vi "HMI CSE1.vi"() -> ()   [LabVIEW 2010]
uses:
  <vilib>/addons/Simulation Interface/_sitctls/sit Indicator Info.ctl
  <vilib>/addons/Simulation Interface/_sitctls/sit Indicator Type.ctl
  <vilib>/addons/Simulation Interface/_sitctls/sit Client Meta Info (v3).ctl
  <vilib>/addons/Simulation Interface/_sitctls/sit MDL Line Item Info.ctl
  <vilib>/addons/Simulation Interface/_sitctls/sit MDL Line Type.ctl
  <vilib>/addons/Simulation Interface/_sitctls/sit Details Settings.ctl
  <vilib>/addons/Simulation Interface/_sitctls/sit Execution Host.ctl
  <vilib>/addons/Simulation Interface/_sitctls/SIT Sim State.ctl
  <vilib>/Utility/inputDevices.llb/closeJoystick.vi
  <vilib>/Utility/inputDevices.llb/joystickAcquire.vi
  <vilib>/addons/Simulation Interface/_sitclient.llb/NI_SIT_sitclient.lvlib
  <vilib>/addons/Simulation Interface/_sitctls/NI_SIT_sitctls.lvlib
  <vilib>/ptbypt/NI_PtbyPt.lvlib
  <vilib>/picture/3D Picture Control/NI_3D Picture Control.lvlib
panel:
  out "Navigation eta yaw":dbl
  out "Navigation eta sway":dbl
  out "Navigation eta surge":dbl
  out "Plant u5":dbl
  out "Plant u4":dbl
  out "Plant u3":dbl
  out "Plant u2":dbl
  out "Plant u1":dbl
  out "DP eta Psi deg":dbl
  out "DP eta E":dbl
  out "DP eta N":dbl
  out "DP eta_d Psi deg":dbl
  out "DP eta_d E":dbl
  out "DP eta_d N":dbl
  in  "Enabler Nothing":bool
  in  "Enable Linear Simulator":bool
  in  "Control Input Selector":enum32{"OK Button 4", "OK Button 5"}(radio)
  in  "MODE":T1(radio)=enum."OK Button 4"
  in  "Enable CSE1 actuator":bool
  in  "SIT_RVE":bool
  in  "SIT_Remap":bool
  in  "SIT_Details":bool
  in  "SIT_Stop":bool
  in  "SIT_Pause":bool
  in  "SIT_Run":bool
  in  "SIT_stopVI":bool
  out "SIT_Status":string
  in  "Tab Front Pannel":T2(tab)
  out "Port VSP Direction":dbl(knob) scale=0.0..360.0
  out "Starboard VSP Direction":dbl(knob) scale=0.0..360.0
  in  "Precision  VSP Speed limit":dbl
  in  "Precision u5":dbl
  in  "Precision u4":dbl
  in  "Precision u3":dbl
  in  "Precision u2":dbl
  in  "Precision u1":dbl
  out "Slide BT red":dbl(slide)
  out "Slide BT green":dbl(slide) scale=0.0..1.0
  out "Magnitude Pitch Starboard VSP":dbl(knob) scale=0.0..1.0
  out "Magnitude Pitch Port VSP":dbl(knob) scale=0.0..1.0
  out "Direction Starboard VSP":cluster{dbl, dbl}(knob)={0.0, -90.87174020086496} scale=180.0..-180.0
  out "Direction Port VSP":cluster{dbl, dbl}(knob)={0.0, 56.36157481708119} scale=180.0..-180.0
  in  "Precision BT Power limit":dbl
  in  "VSP Slide Speed":dbl(slide) min=-1.0 max=1.0 step=0.05 scale=-1.0..1.0 scale format="%#_2g"
  in  "BT Slide Power Limiter":dbl(slide) min=0.0 max=1.0 step=0.1 scale=-1.0..1.0
  in  "Left Y":dbl(slide) scale=-35860.0..35860.0
  in  "Left X":dbl(slide) scale=-35860.0..35860.0
  in  "Right X":dbl(slide) scale=-35860.0..35860.0
  in  "Right Y":dbl(slide) scale=-35860.0..35860.0
  out "Servo Battery":dbl(knob) scale=0.0..8.0
  out "Bowthruster Battery":dbl(knob) scale=0.0..8.0
  out "Main Battery":dbl(knob) scale=0.0..18.0
  out "Left Joystick":bool
  out "Right Joystick":bool
  out "Direction Up":bool
  out "Direction Right":bool
  out "Direction Down":bool
  out "Direction Left":bool
  out "L2 Button":bool
  out "R2 Button":bool
  out "Triangle Button":bool
  out "Circle Button":bool
  out "X Button":bool
  out "Square Button":bool
  out "Joystick Info":T3(array[cluster])
  in  "L2":sgl
  in  "R2":sgl
  out "Plot s":waveform(dbl)[](graph)
  out "Plot q_y":waveform(dbl)[](graph)
  out "Plot q_x":waveform(dbl)[](graph)
  in  "Tab Path":enum32{"Path", "Page 2"}(tab)
  in  "Enable path guidance":bool
  in  "u_d [m/s]":dbl
  out "Path psi_d":dbl
  out "Path y_d":dbl
  out "Path x_d":dbl
  in  "Show Path Marker":bool
  in  "my":dbl
  in  "Delta":dbl
  in  "x_2":dbl
  in  "y_2":dbl
  in  "x_1":dbl
  in  "y_1":dbl
  in  "Tab Plants":enum32{"eta", "Qualisys", "Linear Simulator"}(tab)
  in  "Tab eta":enum32{"Navigation output", "Qualisys"}(tab)
  out "Iceberg yaw":dbl
  out "Iceberg pitch":dbl
  out "Iceberg roll":dbl
  out "Iceberg z-position":dbl
  out "Iceberg y-position":dbl
  out "Iceberg x-position":dbl
  out "CSE1 yaw [rad]":dbl
  out "CSE1 pitch [rad]":dbl
  out "CSE1 roll [rad]":dbl
  out "CSE1 z-position [m]":dbl
  out "CSE1 y-position [m]":dbl
  out "CSE1 x-position [m]":dbl
  out "QS yaw [rad]":dbl
  out "QS pitch [rad]":dbl
  out "QS roll [rad]":dbl
  out "QS z-position [m]":dbl
  out "QS y-position [m]":dbl
  out "QS x-position [m]":dbl
  in  "Show CSEI":bool
  in  "Show Iceberg":bool
  out "QTM In9":dbl
  out "QTM In8":dbl
  out "QTM In7":dbl
  out "QTM In6":dbl
  out "QTM In5":dbl
  out "QTM In4":dbl
  out "QTM In3":dbl
  out "QTM In2":dbl
  out "QTM In1":dbl
  out "LS nu_yaw_hil":dbl
  out "LS nu_sway_hil":dbl
  out "LS nu_surge_hil":dbl
  out "LS etadot_yaw_hil":dbl
  out "LS etadot_sway_hil":dbl
  out "LS etadot_surge_hil":dbl
  out "LS eta_yaw_hil":dbl
  out "LS eta_sway_hil":dbl
  out "LS  eta_surge_hil":dbl
  in  "LS r_0":dbl
  in  "LS v_0":dbl
  in  "LS u_0":dbl
  in  "LS psi_0":dbl
  in  "LS y_0":dbl
  in  "LS x_0":dbl
  in  "Button Reset Linear Simulator Integrator":bool
  in  "Reset Linear Simulator integrator":dbl
  in  "Tab Control system":T4(tab)
  in  "DP Wave Filter":bool
  in  "DP eta_d LPF":bool
  in  "DP K_d Scale":dbl(slide) min=0.0 max=5.0 step=0.25 scale=0.0..5.0
  in  "DP K_i Scale":dbl(slide) min=0.0 max=5.0 step=0.25 scale=0.0..5.0
  in  "DP K_p Scale":dbl(slide) min=0.0 max=10.0 step=0.5 scale=0.0..10.0
  in  "DP eta_d_N [m]":dbl
  in  "DP eta_d_E [m]":dbl
  in  "Button Reset DP Integrator.":bool
  in  "DP eta_d_Psi [deg]":dbl(knob) scale=0.0..360.0 scale format="%#.3p"
  out "Ind eta_d_Psi [rad]":dbl format="%#_2g"
  in  "Reset DP Integrator":dbl
  in  "Show DP Marker":bool
  in  "LgV2 q_y0":dbl
  in  "LgV2 q_x0":dbl
  in  "LgV2 s_0":dbl
  in  "LgV2 lambda":dbl
  in  "LgV2 Gamma_q Sway":dbl
  in  "LgV2 Gamma_q Surge":dbl
  in  "LgV2 K_d yaw":dbl
  in  "LgV2 K_d Sway":dbl
  in  "LgV2 K_d Surge":dbl
  in  "LgV2 K_i yaw":dbl
  in  "LgV2 K_i Sway":dbl
  in  "LgV2 K_i Surge":dbl
  in  "LgV2 K_p yaw":dbl
  in  "LgV2 K_p Sway":dbl
  in  "LgV2 K_p Surge":dbl
  in  "LgV2 kappa_1":dbl
  in  "Button Reset LgV2 q":bool
  in  "Button Reset LgV2 s":bool
  in  "Reset LgV2 q":dbl
  in  "Reset LgV2 s":dbl
  in  "NLPID q_y0":dbl
  in  "NLPID q_x0":dbl
  in  "NLPID s_0":dbl
  in  "NLPID lambda":dbl
  in  "NLPID Gamma_q Sway":dbl
  in  "NLPID Gamma_q Surge":dbl
  in  "NLPID K_d yaw":dbl
  in  "NLPID K_d Sway":dbl
  in  "NLPID K_d Surge":dbl
  in  "NLPID K_i yaw":dbl
  in  "NLPID K_i Sway":dbl
  in  "NLPID K_i Surge":dbl
  in  "NLPID K_p yaw":dbl
  in  "NLPID K_p Sway":dbl
  in  "NLPID K_p Surge":dbl
  in  "Button Reset NLPID s":bool
  in  "Button Reset NLPID q":bool
  in  "Reset NLPID s":dbl
  in  "Reset NLPID q":dbl
  out "3D Picture":refnum<vi>(3d-picture)
  in  "Tab Reg plots":enum32{"DP", "Page 2"}(tab)
  out "DP Reponse N":cluster{"Value":dbl, "Value":dbl}(graph)
  out "DP Error N":waveform(dbl)[](graph)
  out "DP Error E":waveform(dbl)[](graph)
  out "DP Error Psi":waveform(dbl)[](graph)
  out "DP Reponse Psi":cluster{"Value":dbl, "Value":dbl}(graph)
  out "DP Response E":cluster{"Value":dbl, "Value":dbl}(graph)
  in  "Tab Command":enum32{"DP", "Page 2"}(tab)
  out "DP tau surge":waveform(dbl)[](graph)
  out "DP tau sway":waveform(dbl)[](graph)
  out "DP tau yaw":waveform(dbl)[](graph)
  out "DP u_1":waveform(dbl)[](graph)
  out "DP u_2":waveform(dbl)[](graph)
  out "DP u_3":waveform(dbl)[](graph)
  out "DP u_4":waveform(dbl)[](graph)
  out "DP u_5":waveform(dbl)[](graph)
  in  "SIT_Meta_Info":T5
  in  "SIT_Indicator_Indices":T10[](array[typedef])=[{"Indicator Index"=0, "Number of Signals"=1, "Indicator Type"=enum."Knob"}, {"Indicator Index"=-1, "Number of Signals"=0, "Indicator Type"=enum."Digital"}, {"Indicator Index"=-1, "Number of Signals"=0, "Indicator Type"=enum."Digital"}, {"Indicator Index"=3, "Number of Signals"=1, "Indicator Type"=enum."Digital"}, {"Indicator Index"=4, "Number of Signals"=1, "Indicator Type"=enum."Digital"}, {"Indicator Index"=5, "Number of Signals"=1, "Indicator Type"=enum."Digital"}, {"Indicator Index"=-1, "Number of Signals"=0, "Indicator Type"=enum."Digital"}, {"Indicator Index"=7, "Number of Signals"=1, "Indicator Type"=enum."WaveformChart"}, {"Indicator Index"=8, "Number of Signals"=1, "Indicator Type"=enum."WaveformChart"}, {"Indicator Index"=9, "Number of Signals"=1, "Indicator Type"=enum."WaveformChart"}, {"Indicator Index"=10, "Number of Signals"=1, "Indicator Type"=enum."Digital"}, {"Indicator Index"=11, "Number of Signals"=1, "Indicator Type"=enum."Digital"}, {"Indicator Index"=12, "Number of Signals"=1, "Indicator Type"=enum."Digital"}, {"Indicator Index"=13, "Number of Signals"=1, "Indicator Type"=enum."Digital"}, {"Indicator Index"=14, "Number of Signals"=1, "Indicator Type"=enum."Digital"}, {"Indicator Index"=15, "Number of Signals"=1, "Indicator Type"=enum."Digital"}, {"Indicator Index"=16, "Number of Signals"=1, "Indicator Type"=enum."WaveformChart"}, {"Indicator Index"=17, "Number of Signals"=1, "Indicator Type"=enum."WaveformChart"}, {"Indicator Index"=18, "Number of Signals"=1, "Indicator Type"=enum."WaveformChart"}, {"Indicator Index"=19, "Number of Signals"=1, "Indicator Type"=enum."WaveformChart"}, {"Indicator Index"=20, "Number of Signals"=1, "Indicator Type"=enum."WaveformChart"}, {"Indicator Index"=21, "Number of Signals"=1, "Indicator Type"=enum."WaveformChart"}, {"Indicator Index"=22, "Number of Signals"=1, "Indicator Type"=enum."WaveformChart"}, {"Indicator Index"=23, "Number of Signals"=1, "Indicator Type"=enum."WaveformChart"}, {"Indicator Index"=-1, "Number of Signals"=0, "Indicator Type"=enum."Knob"}, {"Indicator Index"=-1, "Number of Signals"=0, "Indicator Type"=enum."Knob"}, {"Indicator Index"=-1, "Number of Signals"=0, "Indicator Type"=enum."Digital"}, {"Indicator Index"=-1, "Number of Signals"=0, "Indicator Type"=enum."Digital"}, {"Indicator Index"=28, "Number of Signals"=1, "Indicator Type"=enum."Digital"}, {"Indicator Index"=29, "Number of Signals"=1, "Indicator Type"=enum."Digital"}, {"Indicator Index"=30, "Number of Signals"=1, "Indicator Type"=enum."Digital"}, {"Indicator Index"=-1, "Number of Signals"=0, "Indicator Type"=enum."Digital"}, {"Indicator Index"=32, "Number of Signals"=1, "Indicator Type"=enum."Digital"}, {"Indicator Index"=33, "Number of Signals"=1, "Indicator Type"=enum."Digital"}, {"Indicator Index"=34, "Number of Signals"=1, "Indicator Type"=enum."Digital"}, {"Indicator Index"=35, "Number of Signals"=1, "Indicator Type"=enum."Digital"}, {"Indicator Index"=36, "Number of Signals"=1, "Indicator Type"=enum."Digital"}, {"Indicator Index"=37, "Number of Signals"=1, "Indicator Type"=enum."Digital"}, {"Indicator Index"=38, "Number of Signals"=1, "Indicator Type"=enum."Digital"}, {"Indicator Index"=39, "Number of Signals"=1, "Indicator Type"=enum."Digital"}, {"Indicator Index"=40, "Number of Signals"=1, "Indicator Type"=enum."Digital"}, {"Indicator Index"=41, "Number of Signals"=1, "Indicator Type"=enum."Knob"}, {"Indicator Index"=42, "Number of Signals"=1, "Indicator Type"=enum."Knob"}, {"Indicator Index"=43, "Number of Signals"=1, "Indicator Type"=enum."Knob"}, {"Indicator Index"=44, "Number of Signals"=1, "Indicator Type"=enum."Digital"}, {"Indicator Index"=45, "Number of Signals"=1, "Indicator Type"=enum."Digital"}, {"Indicator Index"=46, "Number of Signals"=1, "Indicator Type"=enum."Digital"}, {"Indicator Index"=47, "Number of Signals"=1, "Indicator Type"=enum."Digital"}, {"Indicator Index"=48, "Number of Signals"=1, "Indicator Type"=enum."Digital"}, {"Indicator Index"=49, "Number of Signals"=1, "Indicator Type"=enum."Digital"}, {"Indicator Index"=50, "Number of Signals"=1, "Indicator Type"=enum."Digital"}, {"Indicator Index"=51, "Number of Signals"=1, "Indicator Type"=enum."Digital"}, {"Indicator Index"=52, "Number of Signals"=1, "Indicator Type"=enum."Digital"}, {"Indicator Index"=53, "Number of Signals"=1, "Indicator Type"=enum."Digital"}, {"Indicator Index"=54, "Number of Signals"=1, "Indicator Type"=enum."Digital"}, {"Indicator Index"=55, "Number of Signals"=1, "Indicator Type"=enum."WaveformChart"}, {"Indicator Index"=56, "Number of Signals"=1, "Indicator Type"=enum."WaveformChart"}, {"Indicator Index"=57, "Number of Signals"=1, "Indicator Type"=enum."WaveformChart"}, {"Indicator Index"=58, "Number of Signals"=1, "Indicator Type"=enum."Knob"}, {"Indicator Index"=59, "Number of Signals"=1, "Indicator Type"=enum."Digital"}, {"Indicator Index"=60, "Number of Signals"=1, "Indicator Type"=enum."Digital"}, {"Indicator Index"=61, "Number of Signals"=1, "Indicator Type"=enum."Digital"}, {"Indicator Index"=62, "Number of Signals"=1, "Indicator Type"=enum."Digital"}, {"Indicator Index"=63, "Number of Signals"=1, "Indicator Type"=enum."Digital"}, {"Indicator Index"=64, "Number of Signals"=1, "Indicator Type"=enum."Digital"}, {"Indicator Index"=65, "Number of Signals"=1, "Indicator Type"=enum."Digital"}, {"Indicator Index"=66, "Number of Signals"=1, "Indicator Type"=enum."Digital"}, {"Indicator Index"=67, "Number of Signals"=1, "Indicator Type"=enum."Digital"}, {"Indicator Index"=68, "Number of Signals"=1, "Indicator Type"=enum."Digital"}, {"Indicator Index"=69, "Number of Signals"=1, "Indicator Type"=enum."Digital"}, {"Indicator Index"=70, "Number of Signals"=1, "Indicator Type"=enum."Digital"}, {"Indicator Index"=71, "Number of Signals"=1, "Indicator Type"=enum."Digital"}, {"Indicator Index"=72, "Number of Signals"=1, "Indicator Type"=enum."Digital"}, {"Indicator Index"=73, "Number of Signals"=1, "Indicator Type"=enum."Digital"}, {"Indicator Index"=74, "Number of Signals"=1, "Indicator Type"=enum."Knob"}, {"Indicator Index"=75, "Number of Signals"=1, "Indicator Type"=enum."Slide"}, {"Indicator Index"=76, "Number of Signals"=1, "Indicator Type"=enum."Slide"}, {"Indicator Index"=77, "Number of Signals"=1, "Indicator Type"=enum."Knob"}]
  # "MODE"
  # "Controller Input Selector"
  # "TARGET"
  # "Model Controls"
  # "Precision control"
  # "Bowthruster"
  # "VSP Speed"
  # "VSP speed = 1\n\nStarboard VSP\nMax Speed  ClockWise\n\nPort VSP \nMax Speed CounterClockWise"
  # "VSP Speed = -1\n\nStarboard VSP \nMax Speed CounterClockWise\n\nPort VSP\nMax Speed ClockWise"
  # "Port VSP pitch"
  # "Starboard VSP pitch"
  # "Bow Thruster Power Limit"
  # "Max Power"
  # "Max Power"
  # "No Power"
  # "PS3 Joysticks"
  # "Increase BT power limit"
  # "Increase VSP speed"
  # "Decrease BT power limit"
  # "Decrease VSP speed"
  # "Port VSP\n(surge/sway force setpoint)"
  # "Starboard VSP"
  # "C/S Enterprise I"
  # "Toggle visibility"
  # "Iceberg"
  # "Toggle visibility"
  # "Initial eta"
  # "Initial nu"
  # "DP controller gains"
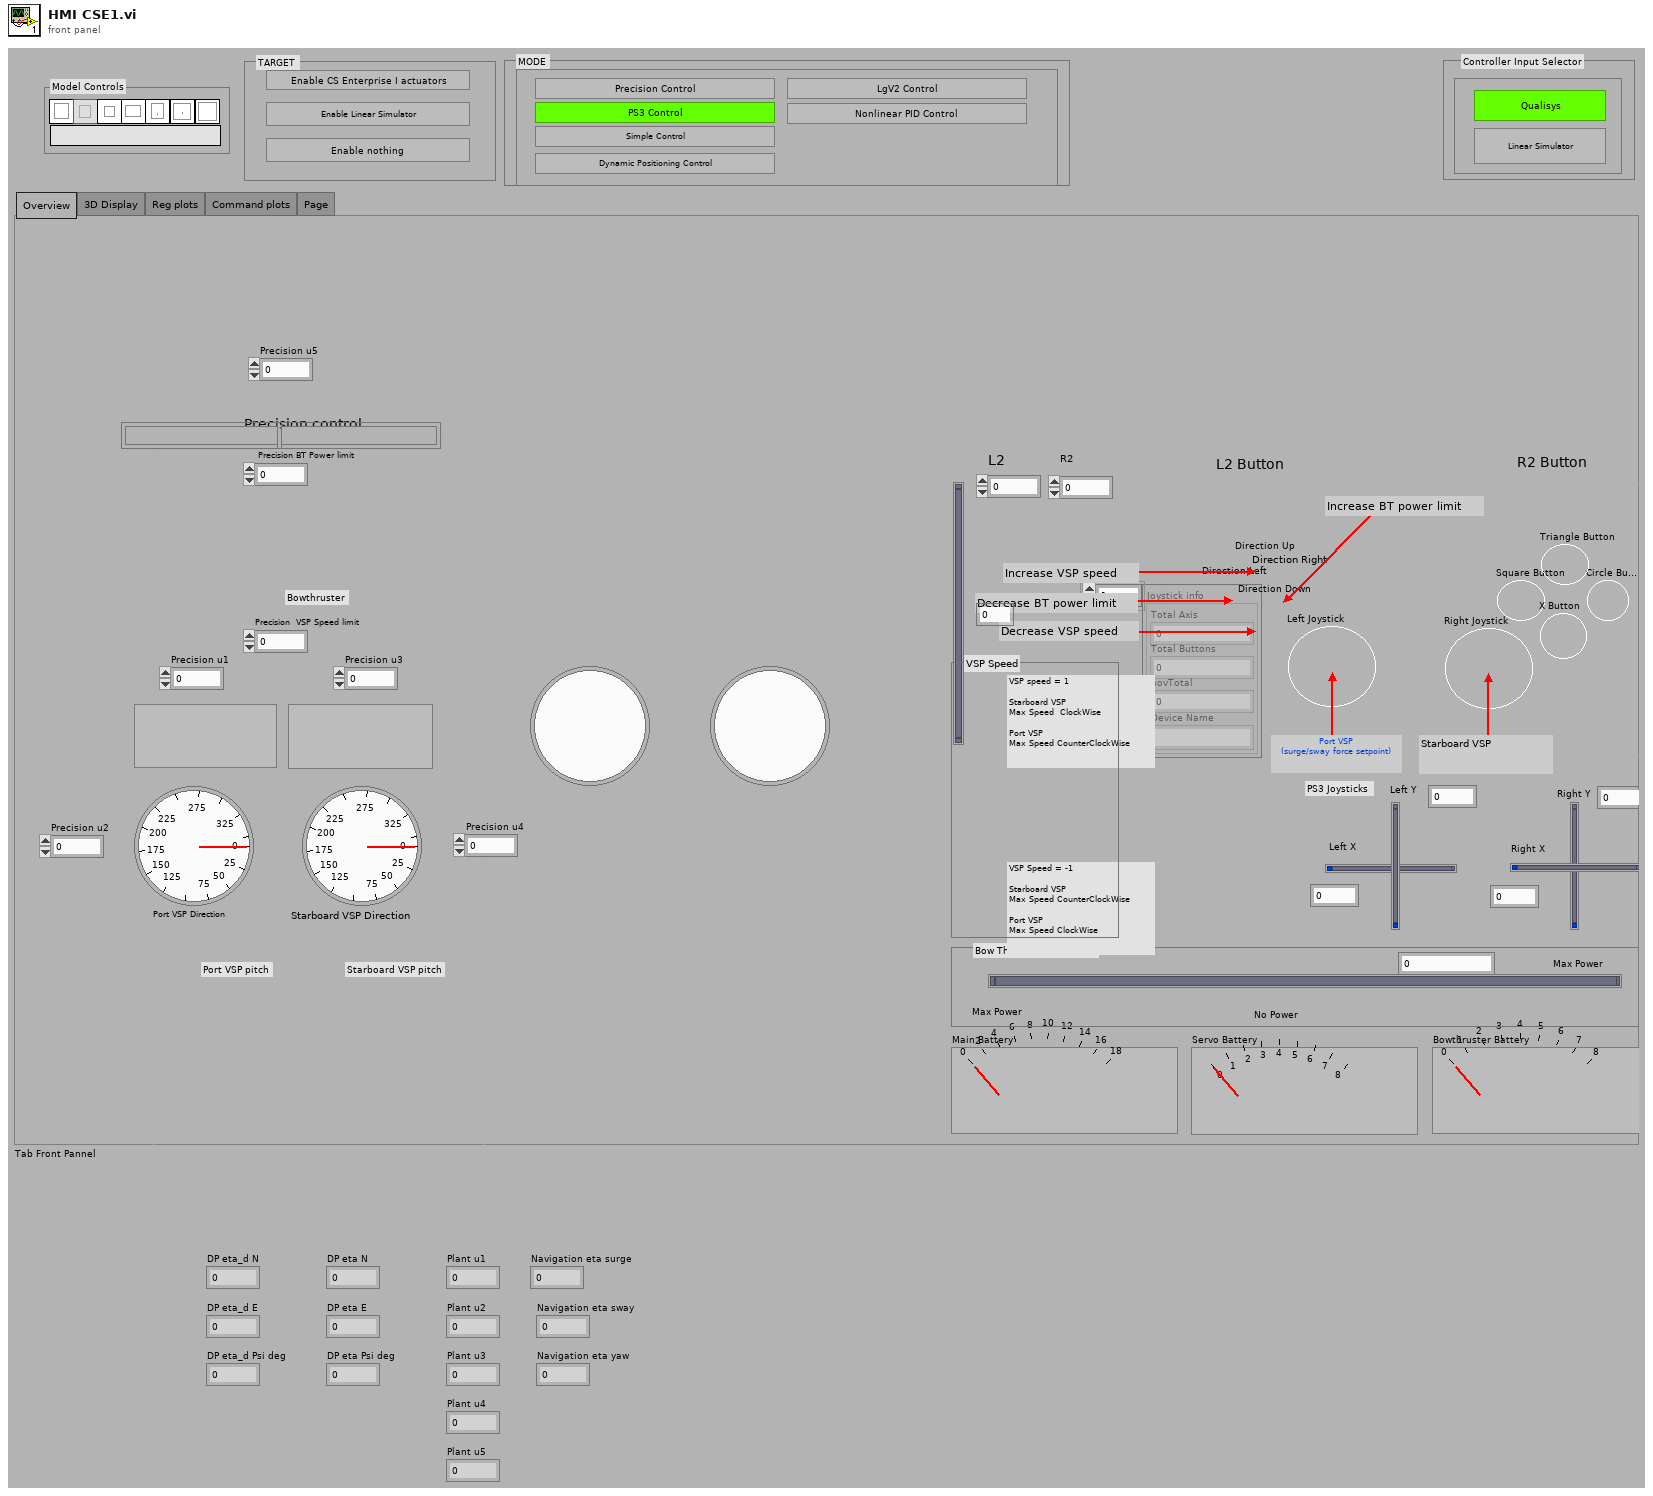
[diagram p1: front panel]
types:
  T1 = enum32{"Radio Selection 4", "OK Button 4", "OK Button 5", "OK Button 6", "Radio Selection 5", "Radio Selection 6"}
  T2 = enum32{"Overview", "3D Display", "Reg plots", "Command plots", "Page"}
  T3 = cluster{"Total Axis":u32, "Total Buttons":u32, "povTotal":u32, "Device Name":string}[]
  T4 = enum32{"DP Control", "LgV2 Control", "NLPID control"}
  T5 = typedef "NI_SIT_sitctls.lvlib/sit Client Meta Info (v3).ctl" = cluster{"Simulation IP":string, "Target IP":string, "Host Port":u16, "Model DLL Path":path, "Model File Path":path, "Model Name":string, "Param Tree Info ":T6[], "Signal Tree Info":T6[], "Details Settings":T8, "Client Name":string, "Stored Model Checksum":string, "Buffer Sizes":cluster{"number of signals":u32, "circular buffer size":u32, "num data points":u32}, "Execution Host":T9, "Project Dir":path, "Last MDL":path}
  T6 = typedef "NI_SIT_sitctls.lvlib/sit MDL Line Item Info.ctl" = cluster{"Line Type":T7, "Section Type":string, "Name":string, "Value":string, "Owner Index":i32, "Tree Tag":string, "Child Indices":i32[], "Expanded?":bool, "Destination Block Info":string[]}
  T7 = typedef "NI_SIT_sitctls.lvlib/sit MDL Line Type.ctl" = enum16{"Section Head", "Parameter", "Section End", "Comment"}
  T8 = typedef "NI_SIT_sitctls.lvlib/sit Details Settings.ctl" = cluster{"Halt on Task Overrun?":bool, "Halt on Lost Data?":bool, "Signal Decimation":i32, "Autoscale":bool}
  T9 = typedef "NI_SIT_sitctls.lvlib/sit Execution Host.ctl" = enum32{"Simulation Environment", "RT Target", "Local Driver"}
  T10 = typedef "NI_SIT_sitctls.lvlib/sit Indicator Info.ctl" = cluster{"Indicator Index":i32, "Number of Signals":i32, "Indicator Type":T11}
  T11 = typedef "NI_SIT_sitctls.lvlib/sit Indicator Type.ctl" = enum32{"xxx1", "xxx2", "xxx3", "Generic   ", "Decoration", "Text", "xControl", "ColorBox", "Boolean", "RefNum", "Variant", "Path", "ListBox", "Table", "Array", "Picture", "ActiveXContainer", "Numeric", "Digital", "NamedNumeric", "ColorRamp", "Slide", "GraphOrChart", "WaveformChart", "WaveformGraph", "IntensityChart", "xxx4", "xxx5", "xxx6", "xxx7", "Cluster", "Panel", "Knob", "NumWithScale", "Ring", "Enum", "GObject", "Plot", "Cursor", "NumericText", "Scale", "ColorScale", "GraphScale", "ColorGraphScale", "TypedRefNum", "OldKnobScale", "MCListbox", "WaveformData", "BVTag", "DAQName", "VISAName", "IVIName", "SlideScale"}
  T12 = cluster{"Red":sgl, "Green":sgl, "Blue":sgl, "Alpha":sgl}
  T13 = cluster{"axes total":u32, "buttons total":u32, "pov total":u32, "device name":string}[]
  T14 = typedef "NI_SIT_sitctls.lvlib/sit TCP Conn and Queue.ctl" = cluster{"TCP Connection":refnum<k5>, "Data Queue":refnum<queue>, "Execution Host":T9}
  T15 = typedef "NI_SIT_sitctls.lvlib/sit Client Op Refs.ctl" = cluster{"Conn and Queue":T14, "RunPauseStop Refs":refnum<vi>[], "Control Refs":refnum<vi>[], "Indicator Refs":refnum<vi>[], "Param Info":T16[], "State Queue":refnum<queue>, "Don't Modify Scales?":bool, "Param Info Needs Init?":bool}
  T16 = typedef "NI_SIT_sitctls.lvlib/SIT param info.ctl" = cluster{"paramidx":i32, "ID":string, "paramname":string, "dattype":i32, "Dimensions":i32[], "value":dbl[]}
  T17 = typedef "NI_SIT_sitctls.lvlib/SIT Sim State.ctl" = enum8{"Default", "Idle", "Running", "Paused", "Stopped", "Error"}
  T18 = cluster{"X axis":i32, "Y axis":i32, "Z axis":i32, "X axis rotation":i32, "Y axis rotation":i32, "Z axis rotation":i32, "U axis":i32, "V axis":i32}
  T19 = cluster{"button 1":bool, "button 2":bool, "button 3":bool, "button 4":bool, "button 5":bool, "button 6":bool, "button 7":bool, "button 8":bool, "button 9":bool, "button 10":bool, "button 11":bool, "button 12":bool, "button 13":bool, "button 14":bool, "button 15":bool, "button 16":bool, "button 17":bool, "button 18":bool, "button 19":bool, "button 20":bool, "button 21":bool, "button 22":bool, "button 23":bool, "button 24":bool, "button 25":bool, "button 26":bool, "button 27":bool, "button 28":bool, "button 29":bool, "button 30":bool, "button 31":bool, "button 32":bool}
  T20 = cluster{"pov 1":i32, "pov 2":i32, "pov 3":i32, "pov 4":i32}
  T21 = cluster{"DP eta_d_N [m]":dbl, i32, "DP eta_d_E [m]":dbl}
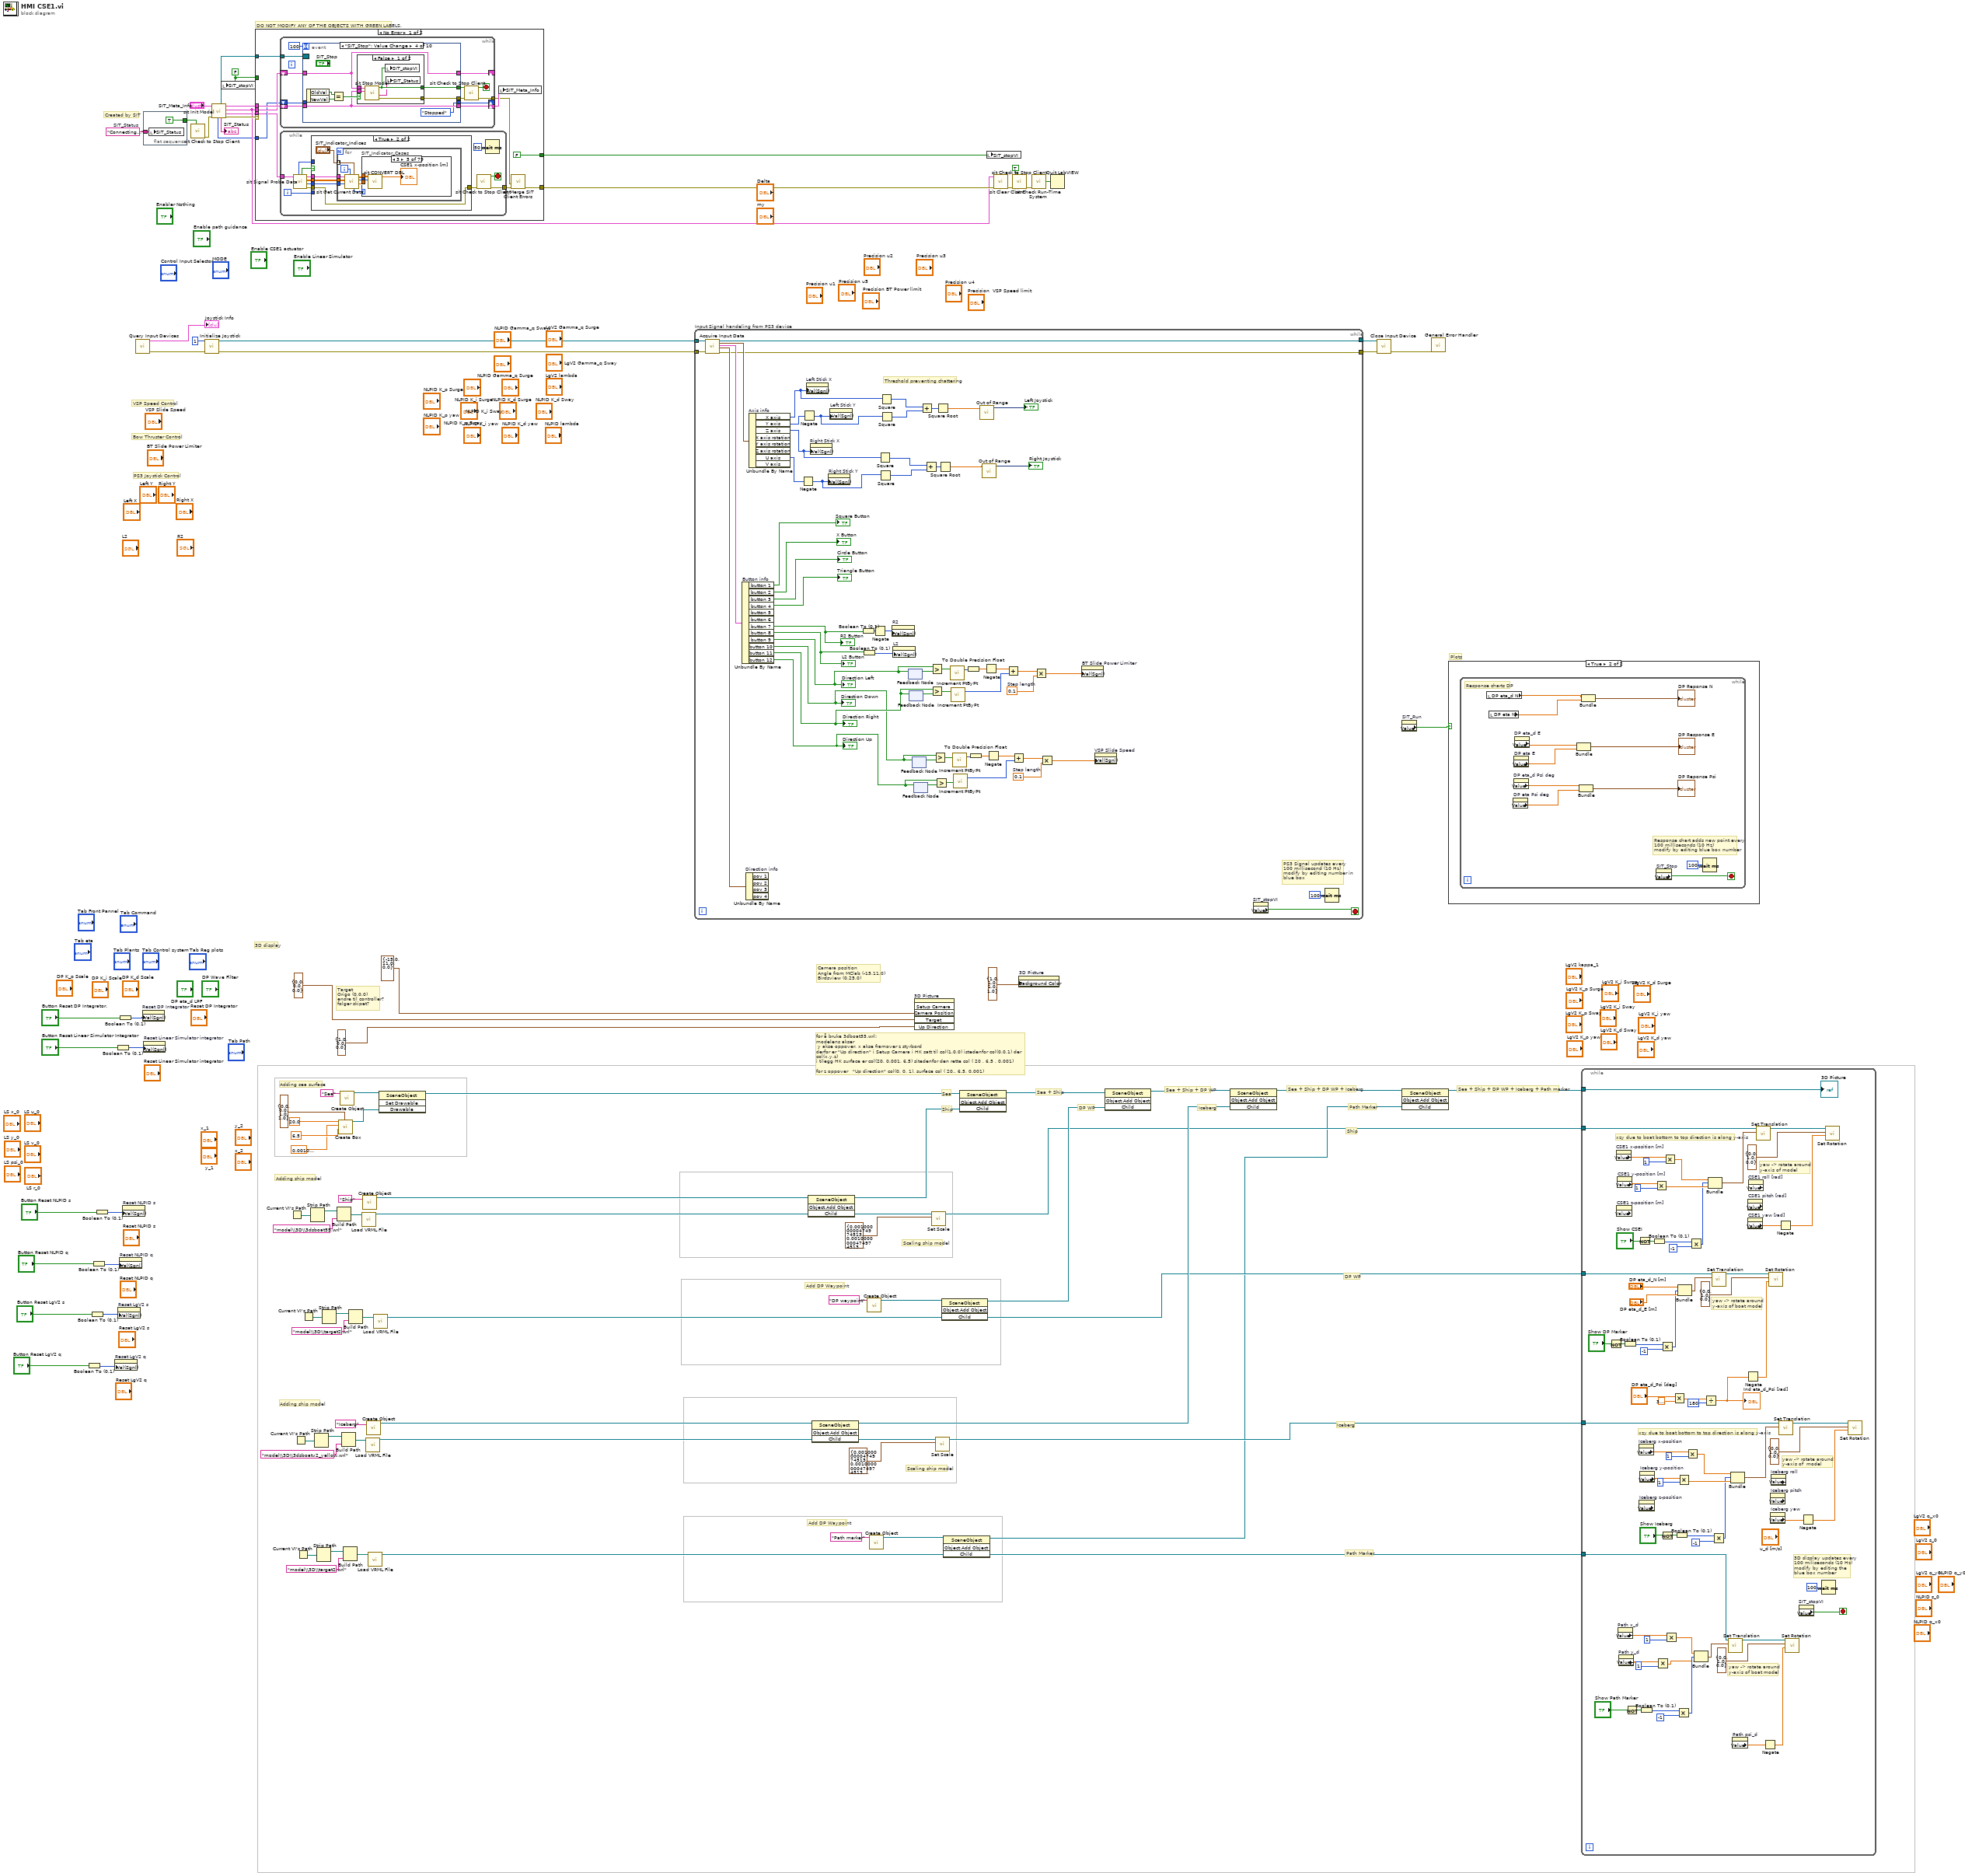
[diagram p0: block diagram]
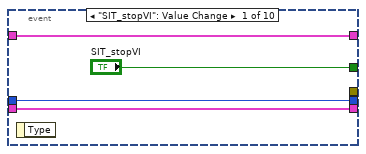
[diagram p3: hidden frame]
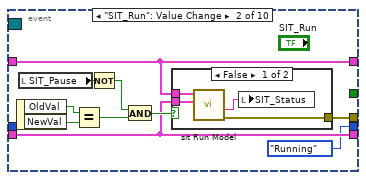
[diagram p4: hidden frame]
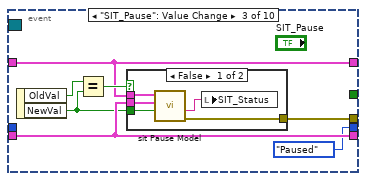
[diagram p6: hidden frame]
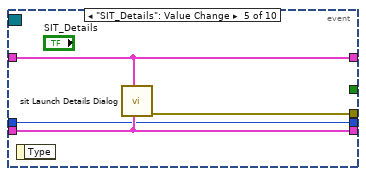
[diagram p9: hidden frame]
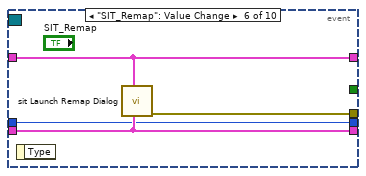
[diagram p10: hidden frame]
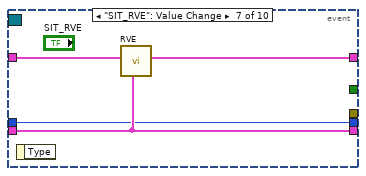
[diagram p11: hidden frame]
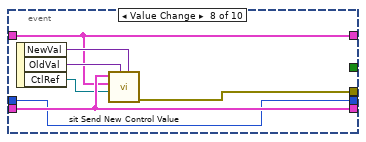
[diagram p12: hidden frame]
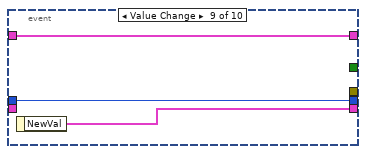
[diagram p13: hidden frame]
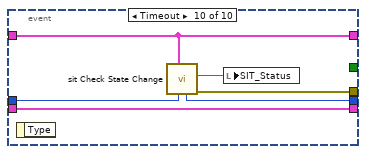
[diagram p14: hidden frame]
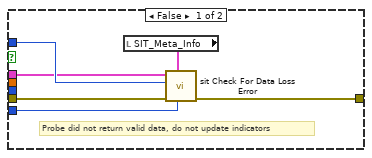
[diagram p15: hidden frame]
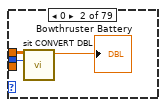
[diagram p17: hidden frame]
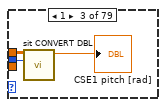
[diagram p18: hidden frame]
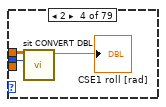
[diagram p19: hidden frame]
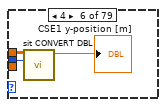
[diagram p20: hidden frame]
diagram:
  w80 = "Connecting..."  # SIT_Status
  w85 = FALSE
  # "Path Marker"
  # "Path Marker"
  # "Sea + Ship + DP WP + Iceberg + Path marker"
  # "Add DP Waypoint"
  # "Plots"
  # "Iceberg"
  # "Iceberg"
  # "Sea + Ship + DP WP + Iceberg"
  # "Scaling ship model"
  # "Adding ship model"
  # "DP WP"
  # "Ship"
  # "3D display"
  # "DP WP"
  # "Target\nOrigo (0,0,0)\nendre til controller?\nfølger skipet?"
  # "Scaling ship model"
  # "Camera position\nAngle from MClab (-15,11,0)\nBirdsview (0,25,0)"
  # "Add DP Waypoint"
  # "Sea + Ship + DP WP"
  # "for å bruke 3dboat55.wrl:\nmodelens akser\n y akse oppover, x akse framover z styrbord\nderfor er \"Up direction\" i Setup Camera i HK satt til col(1,0,0) istedenfor col(0,0,1) der col(x,y,z)\ni tilegg HK surface er col(20, 0.001, 6.5) sitedenfor den rette col ( 20 , 6.5 , 0.001) \n\nfor z oppover   \"Up direction\" col(0, 0, 1), surface col ( 20., 6.5, 0.001)"
  # "Sea + Ship"
  # "Ship"
  # "Sea"
  # "Adding sea surface"
  # "Adding ship model"
  # "VSP Speed Control"
  # "Bow Thruster Control"
  # "Created by SIT"
  # "PS3 Joystick Control"
  # "DO NOT MODIFY ANY OF THE OBJECTS WITH GREEN LABELS."
  n1 = Boolean To (0,1)(Boolean="Button Reset LgV2 q") -> (0, 1=w1:i16)
  n2 = Boolean To (0,1)(Boolean="Button Reset LgV2 s") -> (0, 1=w3:i16)
  n3 = Boolean To (0,1)(Boolean="Button Reset NLPID q") -> (0, 1=w5:i16)
  n4 = Boolean To (0,1)(Boolean="Button Reset NLPID s") -> (0, 1=w7:i16)
  n5 = property on="Reset LgV2 q" class="DigNum (strict)"("Val(Sgnl)"=w1) -> ()  [unwired: 2 in, 2 out]
  n6 = Boolean To (0,1)(Boolean="Button Reset Linear Simulator Integrator") -> (0, 1=w23:i16)
  n7 = Boolean To (0,1)(Boolean="Button Reset DP Integrator.") -> (0, 1=w21:i16)
  n8 = property on="Reset LgV2 s" class="DigNum (strict)"("Val(Sgnl)"=w3) -> ()  [unwired: 2 in, 2 out]
  n9 = property on="Reset NLPID q" class="DigNum (strict)"("Val(Sgnl)"=w5) -> ()  [unwired: 2 in, 2 out]
  n10 = property on="Reset NLPID s" class="DigNum (strict)"("Val(Sgnl)"=w7) -> ()  [unwired: 2 in, 2 out]
  n11 = call <vilib>:"Query Input Devices.vi"() -> ("error out"=w74:errorcluster, "joystick info"=→"Joystick Info":T13)  [unwired: 8 in, 2 out]
  n12 = property on="Reset DP Integrator" class="DigNum (strict)"("Val(Sgnl)"=w21) -> ()  [unwired: 2 in, 2 out]
  n13 = flat-sequence {
    tunnel: [TRUE ("Clear Item?")] -> w89
    tunnel: w80 -> [w96]
    frame #0 {
      n14 = local write "SIT_Status"(w96) -> ()
    }
  }
  n15 = property on="Reset Linear Simulator integrator" class="DigNum (strict)"("Val(Sgnl)"=w23) -> ()  [unwired: 2 in, 2 out]
  n16 = call <vilib>:"sit Check to Stop Client.vi"("Reset Stop?"=w89) -> ("error out"=w91:errorcluster)  [unwired: 2 in, 8 out]
  n17 = call <vilib>:"Initialize Joystick.vi"("error in (no error)"=w74, "device index"=1) -> ("error out"=w76:errorcluster, "device ID"=w77:refnum<k1>)  [unwired: 8 in]
  n18 = call <vilib>:"sit Init Model.vi"("error in (no error)"=w91, "SIT_Meta_Info in"="SIT_Meta_Info") -> ("error out"=w95:errorcluster, "Conn and Queue"=w82:T14, "SIT Client Op Refs"=w86:T15, "SIT_Meta_Info out"=w93:T5, "Initial State"=→"SIT_Status":string, "Event Registration Refnum"=w94:refnum<event-registration>, "State"=w83:T17)  [unwired: 2 in, 1 out]
  n19 = local write "SIT_stopVI"(w85) -> ()
  n20 = case shown="No Error" w95 {
    selector: w95 -> [_ w484]
    tunnel: w94 -> [w107 _]
    tunnel: w93 -> [w105 w483]
    tunnel: [w101 w484] -> w90
    tunnel: w86 -> [w104 _]
    tunnel: w85 -> [_ _]
    tunnel: [FALSE _] -> w84
    tunnel: w83 -> [w99 _]
    tunnel: w82 -> [w98 _]
    frame No Error {
      n21 = while {
        tunnel: w107 -> [w119]
        tunnel: [w117] -> w100
        shift-right: [w111] -> _
        shift-left: w104 -> [w115]
        shift-right: [w118] -> w106
        shift-left: w105 -> [w116]
        shift-right: [w108] -> _
        shift-left: w99 -> [w109]
        stop <- w110 stop-if-true
        n22 = event shown="[3] \"SIT_Stop\": Value Change" {
          selector: w119 -> [_ _ _ _ _ _ _ _ _ _]
          dyn-events: _ -> [_ _ _ _ _ _ _ _ _ _]
          timeout: 100 -> [_ _ _ _ _ _ _ _ _ _]
          tunnel: ["SIT_stopVI" _ _ w154 _ _ _ _ _ _] -> w112
          tunnel: [_ w129 w141 w153 w166 w170 _ w181 _ w188] -> w113
          tunnel: w116 -> [w122 w127 w142 w155 w165 w169 w173 w180 _ w190]
          tunnel: w115 -> [w120 w128 w143 w156 w164 w167 w174 w176 w183 w189]
          tunnel: [w122 w127 w142 w155 w165 w169 w173 w180 w184 w190] -> w118
          tunnel: [w120 w128 w143 w156 w164 w167 w172 w176 w183 w189] -> w111
          tunnel: [w121 SIT_Sim_State."Running" ("State") SIT_Sim_State."Paused" ("State") SIT_Sim_State."Stopped" ("State") w163 w168 w171 w175 w182 w186] -> w108
          tunnel: w109 -> [w121 _ _ _ w163 w168 w171 w175 w182 w187]
          event "SIT_stopVI": Value Change {
            n23 = event-data() -> ()  [unwired: 2 out]
          }
          event "SIT_Run": Value Change {
            n24 = event-data() -> ("OldVal"=w125:bool, "NewVal"=w126:bool)  [unwired: 1 out]
            n25 = local read "SIT_Pause"() -> (w132:bool)
            n26 = Equal?(x=w125, y=w126) -> (x = y?=w130:bool)
            n27 = Not(x=w132) -> (.not. x?=w133:bool)
            n28 = And(x=w133, y=w130) -> (x .and. y?=w131:bool)
            n29 = case shown="False" w131 {
              tunnel: [w137 _] -> w129
              tunnel: w128 -> [w136 _]
              tunnel: w127 -> [w135 _]
              frame False {
                n30 = call <vilib>:"sit Run Model.vi"("SIT Meta Info"=w135, "SIT Client Op Refs"=w136) -> ("error out"=w137:errorcluster, "Status"=w134:string)  [unwired: 6 in, 2 out]
                n31 = local write "SIT_Status"(w134) -> ()
              }
              frame True {
                # "Ignore value change if it is\nto the same value"
              }
            }
          }
          event "SIT_Pause": Value Change {
            n32 = event-data() -> ("OldVal"=w139:bool, "NewVal"=w140:bool)  [unwired: 1 out]
            n33 = Equal?(x=w139, y=w140) -> (x = y?=w144:bool)
            n34 = case shown="False" w144 {
              tunnel: [w149 _] -> w141
              tunnel: w143 -> [w148 _]
              tunnel: w142 -> [w147 _]
              tunnel: w140 -> [w146 _]
              frame False {
                n35 = call <vilib>:"sit Pause Model.vi"("Pause Button Value"=w146, "SIT Meta Info"=w147, "SIT Client Op Refs"=w148) -> ("error out"=w149:errorcluster, "Status"=w145:string)  [unwired: 3 in, 4 out]
                n36 = local write "SIT_Status"(w145) -> ()
              }
              frame True {
                # "Ignore value change if it is\nto the same value"
              }
            }
          }
          event "SIT_Stop": Value Change {
            n37 = event-data() -> ("OldVal"=w151:bool, "NewVal"=w152:bool)  [unwired: 1 out]
            n38 = Equal?(x=w151, y=w152) -> (x = y?=w157:bool)
            n39 = case shown="False" w157 {
              tunnel: [w162 _] -> w153
              tunnel: [w159 _] -> w154
              tunnel: w155 -> [w161 _]
              tunnel: w156 -> [w160 _]
              frame False {
                n40 = call <vilib>:"sit Stop Model.vi"("SIT Meta Info"=w161, "SIT Client Op Refs"=w160) -> ("error out"=w162:errorcluster, "Status"=w158:string, "Stop VI?"=w159:bool)  [unwired: 4 in, 3 out]
                n41 = local write "SIT_stopVI"(w159) -> ()
                n42 = local write "SIT_Status"(w158) -> ()
              }
              frame True {
                # "Ignore value change if it is\nto the same value"
              }
            }
          }
          event "SIT_Details": Value Change {
            n43 = event-data() -> ()  [unwired: 2 out]
            n44 = call <vilib>:"sit Launch Details Dialog.vi"("SIT Meta Info in"=w165, "SIT Client Op Refs"=w164) -> ("error out"=w166:errorcluster)  [unwired: 1 in, 8 out]
          }
          event "SIT_Remap": Value Change {
            n45 = event-data() -> ()  [unwired: 2 out]
            n46 = call <vilib>:"sit Launch Remap Dialog.vi"("SIT Meta Info in"=w169, "SIT Client Op Refs"=w167) -> ("error out"=w170:errorcluster)  [unwired: 2 in, 7 out]
          }
          event "SIT_RVE": Value Change {
            n47 = event-data() -> ()  [unwired: 2 out]
            n48 = call <vilib>:"RVE.vi"("SIT_Meta_Info"=w173, "SIT Client Op Refs in"=w174) -> ("SIT Client Op Refs out"=w172:T15)  [unwired: 9 out]
          }
          event Value Change {
            n49 = event-data() -> ("NewVal"=w177:variant, "OldVal"=w178:variant, "CtlRef"=w179:refnum<vi>)  [unwired: 1 out]
            n50 = call <vilib>:"sit Send New Control Value.vi"("Control New Value"=w177, "Control Old Value"=w178, "Control Ref"=w179, "SIT Client Op Refs"=w176, "SIT_Meta_Info"=w180) -> ("error out"=w181:errorcluster)  [unwired: 4 in, 2 out]
          }
          event Value Change {
            n51 = event-data() -> ("NewVal"=w184:T5)  [unwired: 1 out]
          }
          event Timeout {
            n52 = event-data() -> ()  [unwired: 2 out]
            n53 = call <vilib>:"sit Check State Change.vi"("Old State in"=w187, "SIT Client Op Refs"=w189) -> ("error out"=w188:errorcluster, "Status String"=w185:string, "New State out"=w186:T17)  [unwired: 7 out]
            n54 = local write "SIT_Status"(w185) -> ()
          }
        }
        n55 = call <vilib>:"sit Check to Stop Client.vi"("error in (no error)"=w113, "User Stop?"=w112) -> ("error out"=w117:errorcluster, "Stop?"=w110:bool)  [unwired: 1 in, 7 out]
      }
      n56 = while "Read Loop" {
        tunnel: [w201] -> w102
        tunnel: w98 -> [w191]
        i -> [w198]
        stop <- w199 stop-if-true
        n57 = call <vilib>:"sit Signal Probe Data.vi"("TCP Conn and Queue"=w191) -> ("error out"=w194:errorcluster, "Dimensions"=w195:i32[], "Raw Data"=w196:dbl[][], "dup TCP Conn and Queue"=w197:T14, "Valid Data?"=w192:bool, "Options out"=w193:u32)  [unwired: 4 in, 1 out]
        n58 = case shown="True" w192 {
          tunnel: w196 -> [_ w212]
          tunnel: w195 -> [_ w211]
          tunnel: w197 -> [w204 w210]
          tunnel: w194 -> [w207 w209]
          tunnel: [w206 w209] -> w200
          tunnel: w193 -> [w208 _]
          tunnel: w198 -> [w205 _]
          frame False {
            # "Probe did not return valid data, do not update indicators"
            n59 = local read "SIT_Meta_Info"() -> (w203:T5)
            n60 = call <vilib>:"sit Check For Data Loss Error.vi"("Iteration"=w205, "SIT Meta Info"=w203, "error in (no error)"=w207, "Options"=w208, "TCP Conn and Queue"=w204) -> ("error out"=w206:errorcluster)  [unwired: 6 out]
          }
          frame True {
            n61 = for {
              tunnel: w212 -> [w222]
              tunnel: "SIT_Indicator_Indices" -> [w218] mode=indexing
              tunnel: w211 -> [w221]
              tunnel: w210 -> [w219]
              i -> [w220]
              n62 = call <vilib>:"sit Get Current Data.vi"("Indicator Index Cluster"=w218, "Iteration"=w220, "Dimensions"=w221, "Raw Data"=w222, "Conn and Queue"=w219) -> ("Timestamps"=w215:dbl[], "Last Row"=w216:i32, "Current Data"=w217:dbl[][], "Indicator Index"=w214:i32)  [unwired: 1 in, 2 out]
              n63 = case "SIT_Indicator_Cases" shown="3" w214 {
                tunnel: w217 -> [_ w225 w228 w231 w234 w237 w240 w243 w247 w252 w257 w261 w264 w267 w270 w273 w276 w280 w285 w290 w295 w300 w305 w310 w315 w318 w320 w323 w326 w329 w332 w335 w338 w341 w344 w347 w350 w353 w356 w359 w362 w365 w368 w371 w374 w377 w380 w383 w386 w389 w392 w395 w398 w401 w404 w407 w411 w416 w421 w425 w428 w431 w434 w437 w440 w443 w446 w449 w452 w455 w458 w461 w464 w467 w470 w473 w476 w479 w482]
                tunnel: w216 -> [_ w224 w227 w230 w233 w236 w239 w242 w246 w251 w256 w260 w263 w266 w269 w272 w275 w279 w284 w289 w294 w299 w304 w309 w314 w317 w319 w322 w325 w328 w331 w334 w337 w340 w343 w346 w349 w352 w355 w358 w361 w364 w367 w370 w373 w376 w379 w382 w385 w388 w391 w394 w397 w400 w403 w406 w410 w415 w420 w424 w427 w430 w433 w436 w439 w442 w445 w448 w451 w454 w457 w460 w463 w466 w469 w472 w475 w478 w481]
                tunnel: w215 -> [_ _ _ _ _ _ _ _ w245 w250 w255 _ _ _ _ _ _ w278 w283 w288 w293 w298 w303 w308 w313 _ _ _ _ _ _ _ _ _ _ _ _ _ _ _ _ _ _ _ _ _ _ _ _ _ _ _ _ _ _ _ w409 w414 w419 _ _ _ _ _ _ _ _ _ _ _ _ _ _ _ _ _ _ _ _]
                frame -1, Default {
                }
                frame 0 {
                  n64 = call <vilib>:"sit CONVERT DBL.vi"("Last Row"=w224, "Raw Data"=w225) -> ("Output"=→"Bowthruster Battery":dbl)  [unwired: 9 in]
                }
                frame 1 {
                  n65 = call <vilib>:"sit CONVERT DBL.vi"("Last Row"=w227, "Raw Data"=w228) -> ("Output"=→"CSE1 pitch [rad]":dbl)  [unwired: 9 in]
                }
                frame 2 {
                  n66 = call <vilib>:"sit CONVERT DBL.vi"("Last Row"=w230, "Raw Data"=w231) -> ("Output"=→"CSE1 roll [rad]":dbl)  [unwired: 9 in]
                }
                frame 3 {
                  n67 = call <vilib>:"sit CONVERT DBL.vi"("Last Row"=w233, "Raw Data"=w234) -> ("Output"=→"CSE1 x-position [m]":dbl)  [unwired: 9 in]
                }
                frame 4 {
                  n68 = call <vilib>:"sit CONVERT DBL.vi"("Last Row"=w236, "Raw Data"=w237) -> ("Output"=→"CSE1 y-position [m]":dbl)  [unwired: 9 in]
                }
                frame 5 {
                  n69 = call <vilib>:"sit CONVERT DBL.vi"("Last Row"=w239, "Raw Data"=w240) -> ("Output"=→"CSE1 yaw [rad]":dbl)  [unwired: 9 in]
                }
                frame 6 {
                  n70 = call <vilib>:"sit CONVERT DBL.vi"("Last Row"=w242, "Raw Data"=w243) -> ("Output"=→"CSE1 z-position [m]":dbl)  [unwired: 9 in]
                }
                frame 7 {
                  n71 = call <vilib>:"sit CONVERT WaveformChart.vi"("Timestamps"=w245, "Last Row"=w246, "Raw Data"=w247) -> ("Output"=w244:waveform(dbl)[][])  [unwired: 8 in]
                  n72 = for {
                    tunnel: w244 -> [w248] mode=indexing
                    "DP Error E" <- w248
                  }
                }
                frame 8 {
                  n73 = call <vilib>:"sit CONVERT WaveformChart.vi"("Timestamps"=w250, "Last Row"=w251, "Raw Data"=w252) -> ("Output"=w249:waveform(dbl)[][])  [unwired: 8 in]
                  n74 = for {
                    tunnel: w249 -> [w253] mode=indexing
                    "DP Error N" <- w253
                  }
                }
                frame 9 {
                  n75 = call <vilib>:"sit CONVERT WaveformChart.vi"("Timestamps"=w255, "Last Row"=w256, "Raw Data"=w257) -> ("Output"=w254:waveform(dbl)[][])  [unwired: 8 in]
                  n76 = for {
                    tunnel: w254 -> [w258] mode=indexing
                    "DP Error Psi" <- w258
                  }
                }
                frame 10 {
                  n77 = call <vilib>:"sit CONVERT DBL.vi"("Last Row"=w260, "Raw Data"=w261) -> ("Output"=→"DP eta E":dbl)  [unwired: 9 in]
                }
                frame 11 {
                  n78 = call <vilib>:"sit CONVERT DBL.vi"("Last Row"=w263, "Raw Data"=w264) -> ("Output"=→"DP eta N":dbl)  [unwired: 9 in]
                }
                frame 12 {
                  n79 = call <vilib>:"sit CONVERT DBL.vi"("Last Row"=w266, "Raw Data"=w267) -> ("Output"=→"DP eta Psi deg":dbl)  [unwired: 9 in]
                }
                frame 13 {
                  n80 = call <vilib>:"sit CONVERT DBL.vi"("Last Row"=w269, "Raw Data"=w270) -> ("Output"=→"DP eta_d E":dbl)  [unwired: 9 in]
                }
                frame 14 {
                  n81 = call <vilib>:"sit CONVERT DBL.vi"("Last Row"=w272, "Raw Data"=w273) -> ("Output"=→"DP eta_d N":dbl)  [unwired: 9 in]
                }
                frame 15 {
                  n82 = call <vilib>:"sit CONVERT DBL.vi"("Last Row"=w275, "Raw Data"=w276) -> ("Output"=→"DP eta_d Psi deg":dbl)  [unwired: 9 in]
                }
                frame 16 {
                  n83 = call <vilib>:"sit CONVERT WaveformChart.vi"("Timestamps"=w278, "Last Row"=w279, "Raw Data"=w280) -> ("Output"=w277:waveform(dbl)[][])  [unwired: 8 in]
                  n84 = for {
                    tunnel: w277 -> [w281] mode=indexing
                    "DP tau surge" <- w281
                  }
                }
                frame 17 {
                  n85 = call <vilib>:"sit CONVERT WaveformChart.vi"("Timestamps"=w283, "Last Row"=w284, "Raw Data"=w285) -> ("Output"=w282:waveform(dbl)[][])  [unwired: 8 in]
                  n86 = for {
                    tunnel: w282 -> [w286] mode=indexing
                    "DP tau sway" <- w286
                  }
                }
                frame 18 {
                  n87 = call <vilib>:"sit CONVERT WaveformChart.vi"("Timestamps"=w288, "Last Row"=w289, "Raw Data"=w290) -> ("Output"=w287:waveform(dbl)[][])  [unwired: 8 in]
                  n88 = for {
                    tunnel: w287 -> [w291] mode=indexing
                    "DP tau yaw" <- w291
                  }
                }
                frame 19 {
                  n89 = call <vilib>:"sit CONVERT WaveformChart.vi"("Timestamps"=w293, "Last Row"=w294, "Raw Data"=w295) -> ("Output"=w292:waveform(dbl)[][])  [unwired: 8 in]
                  n90 = for {
                    tunnel: w292 -> [w296] mode=indexing
                    "DP u_1" <- w296
                  }
                }
                frame 20 {
                  n91 = call <vilib>:"sit CONVERT WaveformChart.vi"("Timestamps"=w298, "Last Row"=w299, "Raw Data"=w300) -> ("Output"=w297:waveform(dbl)[][])  [unwired: 8 in]
                  n92 = for {
                    tunnel: w297 -> [w301] mode=indexing
                    "DP u_2" <- w301
                  }
                }
                frame 21 {
                  n93 = call <vilib>:"sit CONVERT WaveformChart.vi"("Timestamps"=w303, "Last Row"=w304, "Raw Data"=w305) -> ("Output"=w302:waveform(dbl)[][])  [unwired: 8 in]
                  n94 = for {
                    tunnel: w302 -> [w306] mode=indexing
                    "DP u_3" <- w306
                  }
                }
                frame 22 {
                  n95 = call <vilib>:"sit CONVERT WaveformChart.vi"("Timestamps"=w308, "Last Row"=w309, "Raw Data"=w310) -> ("Output"=w307:waveform(dbl)[][])  [unwired: 8 in]
                  n96 = for {
                    tunnel: w307 -> [w311] mode=indexing
                    "DP u_4" <- w311
                  }
                }
                frame 23 {
                  n97 = call <vilib>:"sit CONVERT WaveformChart.vi"("Timestamps"=w313, "Last Row"=w314, "Raw Data"=w315) -> ("Output"=w312:waveform(dbl)[][])  [unwired: 8 in]
                  n98 = for {
                    tunnel: w312 -> [w316] mode=indexing
                    "DP u_5" <- w316
                  }
                }
                frame 24 {
                  n99 = call <vilib>:"sit CONVERT DBL.vi"("Last Row"=w317, "Raw Data"=w318) -> ()  [unwired: 9 in, 1 out]
                }
                frame 25 {
                  n100 = call <vilib>:"sit CONVERT DBL.vi"("Last Row"=w319, "Raw Data"=w320) -> ()  [unwired: 9 in, 1 out]
                }
                frame 26 {
                  n101 = call <vilib>:"sit CONVERT DBL.vi"("Last Row"=w322, "Raw Data"=w323) -> ("Output"=→"Iceberg pitch":dbl)  [unwired: 9 in]
                }
                frame 27 {
                  n102 = call <vilib>:"sit CONVERT DBL.vi"("Last Row"=w325, "Raw Data"=w326) -> ("Output"=→"Iceberg roll":dbl)  [unwired: 9 in]
                }
                frame 28 {
                  n103 = call <vilib>:"sit CONVERT DBL.vi"("Last Row"=w328, "Raw Data"=w329) -> ("Output"=→"Iceberg x-position":dbl)  [unwired: 9 in]
                }
                frame 29 {
                  n104 = call <vilib>:"sit CONVERT DBL.vi"("Last Row"=w331, "Raw Data"=w332) -> ("Output"=→"Iceberg y-position":dbl)  [unwired: 9 in]
                }
                frame 30 {
                  n105 = call <vilib>:"sit CONVERT DBL.vi"("Last Row"=w334, "Raw Data"=w335) -> ("Output"=→"Iceberg yaw":dbl)  [unwired: 9 in]
                }
                frame 31 {
                  n106 = call <vilib>:"sit CONVERT DBL.vi"("Last Row"=w337, "Raw Data"=w338) -> ("Output"=→"Iceberg z-position":dbl)  [unwired: 9 in]
                }
                frame 32 {
                  n107 = call <vilib>:"sit CONVERT DBL.vi"("Last Row"=w340, "Raw Data"=w341) -> ("Output"=→"LS  eta_surge_hil":dbl)  [unwired: 9 in]
                }
                frame 33 {
                  n108 = call <vilib>:"sit CONVERT DBL.vi"("Last Row"=w343, "Raw Data"=w344) -> ("Output"=→"LS eta_sway_hil":dbl)  [unwired: 9 in]
                }
                frame 34 {
                  n109 = call <vilib>:"sit CONVERT DBL.vi"("Last Row"=w346, "Raw Data"=w347) -> ("Output"=→"LS eta_yaw_hil":dbl)  [unwired: 9 in]
                }
                frame 35 {
                  n110 = call <vilib>:"sit CONVERT DBL.vi"("Last Row"=w349, "Raw Data"=w350) -> ("Output"=→"LS etadot_surge_hil":dbl)  [unwired: 9 in]
                }
                frame 36 {
                  n111 = call <vilib>:"sit CONVERT DBL.vi"("Last Row"=w352, "Raw Data"=w353) -> ("Output"=→"LS etadot_sway_hil":dbl)  [unwired: 9 in]
                }
                frame 37 {
                  n112 = call <vilib>:"sit CONVERT DBL.vi"("Last Row"=w355, "Raw Data"=w356) -> ("Output"=→"LS etadot_yaw_hil":dbl)  [unwired: 9 in]
                }
                frame 38 {
                  n113 = call <vilib>:"sit CONVERT DBL.vi"("Last Row"=w358, "Raw Data"=w359) -> ("Output"=→"LS nu_surge_hil":dbl)  [unwired: 9 in]
                }
                frame 39 {
                  n114 = call <vilib>:"sit CONVERT DBL.vi"("Last Row"=w361, "Raw Data"=w362) -> ("Output"=→"LS nu_sway_hil":dbl)  [unwired: 9 in]
                }
                frame 40 {
                  n115 = call <vilib>:"sit CONVERT DBL.vi"("Last Row"=w364, "Raw Data"=w365) -> ("Output"=→"LS nu_yaw_hil":dbl)  [unwired: 9 in]
                }
                frame 41 {
                  n116 = call <vilib>:"sit CONVERT DBL.vi"("Last Row"=w367, "Raw Data"=w368) -> ("Output"=→"Magnitude Pitch Port VSP":dbl)  [unwired: 9 in]
                }
                frame 42 {
                  n117 = call <vilib>:"sit CONVERT DBL.vi"("Last Row"=w370, "Raw Data"=w371) -> ("Output"=→"Magnitude Pitch Starboard VSP":dbl)  [unwired: 9 in]
                }
                frame 43 {
                  n118 = call <vilib>:"sit CONVERT DBL.vi"("Last Row"=w373, "Raw Data"=w374) -> ("Output"=→"Main Battery":dbl)  [unwired: 9 in]
                }
                frame 44 {
                  n119 = call <vilib>:"sit CONVERT DBL.vi"("Last Row"=w376, "Raw Data"=w377) -> ("Output"=→"Navigation eta surge":dbl)  [unwired: 9 in]
                }
                frame 45 {
                  n120 = call <vilib>:"sit CONVERT DBL.vi"("Last Row"=w379, "Raw Data"=w380) -> ("Output"=→"Navigation eta sway":dbl)  [unwired: 9 in]
                }
                frame 46 {
                  n121 = call <vilib>:"sit CONVERT DBL.vi"("Last Row"=w382, "Raw Data"=w383) -> ("Output"=→"Navigation eta yaw":dbl)  [unwired: 9 in]
                }
                frame 47 {
                  n122 = call <vilib>:"sit CONVERT DBL.vi"("Last Row"=w385, "Raw Data"=w386) -> ("Output"=→"Path psi_d":dbl)  [unwired: 9 in]
                }
                frame 48 {
                  n123 = call <vilib>:"sit CONVERT DBL.vi"("Last Row"=w388, "Raw Data"=w389) -> ("Output"=→"Path x_d":dbl)  [unwired: 9 in]
                }
                frame 49 {
                  n124 = call <vilib>:"sit CONVERT DBL.vi"("Last Row"=w391, "Raw Data"=w392) -> ("Output"=→"Path y_d":dbl)  [unwired: 9 in]
                }
                frame 50 {
                  n125 = call <vilib>:"sit CONVERT DBL.vi"("Last Row"=w394, "Raw Data"=w395) -> ("Output"=→"Plant u1":dbl)  [unwired: 9 in]
                }
                frame 51 {
                  n126 = call <vilib>:"sit CONVERT DBL.vi"("Last Row"=w397, "Raw Data"=w398) -> ("Output"=→"Plant u2":dbl)  [unwired: 9 in]
                }
                frame 52 {
                  n127 = call <vilib>:"sit CONVERT DBL.vi"("Last Row"=w400, "Raw Data"=w401) -> ("Output"=→"Plant u3":dbl)  [unwired: 9 in]
                }
                frame 53 {
                  n128 = call <vilib>:"sit CONVERT DBL.vi"("Last Row"=w403, "Raw Data"=w404) -> ("Output"=→"Plant u4":dbl)  [unwired: 9 in]
                }
                frame 54 {
                  n129 = call <vilib>:"sit CONVERT DBL.vi"("Last Row"=w406, "Raw Data"=w407) -> ("Output"=→"Plant u5":dbl)  [unwired: 9 in]
                }
                frame 55 {
                  n130 = call <vilib>:"sit CONVERT WaveformChart.vi"("Timestamps"=w409, "Last Row"=w410, "Raw Data"=w411) -> ("Output"=w408:waveform(dbl)[][])  [unwired: 8 in]
                  n131 = for {
                    tunnel: w408 -> [w412] mode=indexing
                    "Plot q_x" <- w412
                  }
                }
                frame 56 {
                  n132 = call <vilib>:"sit CONVERT WaveformChart.vi"("Timestamps"=w414, "Last Row"=w415, "Raw Data"=w416) -> ("Output"=w413:waveform(dbl)[][])  [unwired: 8 in]
                  n133 = for {
                    tunnel: w413 -> [w417] mode=indexing
                    "Plot q_y" <- w417
                  }
                }
                frame 57 {
                  n134 = call <vilib>:"sit CONVERT WaveformChart.vi"("Timestamps"=w419, "Last Row"=w420, "Raw Data"=w421) -> ("Output"=w418:waveform(dbl)[][])  [unwired: 8 in]
                  n135 = for {
                    tunnel: w418 -> [w422] mode=indexing
                    "Plot s" <- w422
                  }
                }
                frame 58 {
                  n136 = call <vilib>:"sit CONVERT DBL.vi"("Last Row"=w424, "Raw Data"=w425) -> ("Output"=→"Port VSP Direction":dbl)  [unwired: 9 in]
                }
                frame 59 {
                  n137 = call <vilib>:"sit CONVERT DBL.vi"("Last Row"=w427, "Raw Data"=w428) -> ("Output"=→"QS pitch [rad]":dbl)  [unwired: 9 in]
                }
                frame 60 {
                  n138 = call <vilib>:"sit CONVERT DBL.vi"("Last Row"=w430, "Raw Data"=w431) -> ("Output"=→"QS roll [rad]":dbl)  [unwired: 9 in]
                }
                frame 61 {
                  n139 = call <vilib>:"sit CONVERT DBL.vi"("Last Row"=w433, "Raw Data"=w434) -> ("Output"=→"QS x-position [m]":dbl)  [unwired: 9 in]
                }
                frame 62 {
                  n140 = call <vilib>:"sit CONVERT DBL.vi"("Last Row"=w436, "Raw Data"=w437) -> ("Output"=→"QS y-position [m]":dbl)  [unwired: 9 in]
                }
                frame 63 {
                  n141 = call <vilib>:"sit CONVERT DBL.vi"("Last Row"=w439, "Raw Data"=w440) -> ("Output"=→"QS yaw [rad]":dbl)  [unwired: 9 in]
                }
                frame 64 {
                  n142 = call <vilib>:"sit CONVERT DBL.vi"("Last Row"=w442, "Raw Data"=w443) -> ("Output"=→"QS z-position [m]":dbl)  [unwired: 9 in]
                }
                frame 65 {
                  n143 = call <vilib>:"sit CONVERT DBL.vi"("Last Row"=w445, "Raw Data"=w446) -> ("Output"=→"QTM In1":dbl)  [unwired: 9 in]
                }
                frame 66 {
                  n144 = call <vilib>:"sit CONVERT DBL.vi"("Last Row"=w448, "Raw Data"=w449) -> ("Output"=→"QTM In2":dbl)  [unwired: 9 in]
                }
                frame 67 {
                  n145 = call <vilib>:"sit CONVERT DBL.vi"("Last Row"=w451, "Raw Data"=w452) -> ("Output"=→"QTM In3":dbl)  [unwired: 9 in]
                }
                frame 68 {
                  n146 = call <vilib>:"sit CONVERT DBL.vi"("Last Row"=w454, "Raw Data"=w455) -> ("Output"=→"QTM In4":dbl)  [unwired: 9 in]
                }
                frame 69 {
                  n147 = call <vilib>:"sit CONVERT DBL.vi"("Last Row"=w457, "Raw Data"=w458) -> ("Output"=→"QTM In5":dbl)  [unwired: 9 in]
                }
                frame 70 {
                  n148 = call <vilib>:"sit CONVERT DBL.vi"("Last Row"=w460, "Raw Data"=w461) -> ("Output"=→"QTM In6":dbl)  [unwired: 9 in]
                }
                frame 71 {
                  n149 = call <vilib>:"sit CONVERT DBL.vi"("Last Row"=w463, "Raw Data"=w464) -> ("Output"=→"QTM In7":dbl)  [unwired: 9 in]
                }
                frame 72 {
                  n150 = call <vilib>:"sit CONVERT DBL.vi"("Last Row"=w466, "Raw Data"=w467) -> ("Output"=→"QTM In8":dbl)  [unwired: 9 in]
                }
                frame 73 {
                  n151 = call <vilib>:"sit CONVERT DBL.vi"("Last Row"=w469, "Raw Data"=w470) -> ("Output"=→"QTM In9":dbl)  [unwired: 9 in]
                }
                frame 74 {
                  n152 = call <vilib>:"sit CONVERT DBL.vi"("Last Row"=w472, "Raw Data"=w473) -> ("Output"=→"Servo Battery":dbl)  [unwired: 9 in]
                }
                frame 75 {
                  n153 = call <vilib>:"sit CONVERT DBL.vi"("Last Row"=w475, "Raw Data"=w476) -> ("Output"=→"Slide BT green":dbl)  [unwired: 9 in]
                }
                frame 76 {
                  n154 = call <vilib>:"sit CONVERT DBL.vi"("Last Row"=w478, "Raw Data"=w479) -> ("Output"=→"Slide BT red":dbl)  [unwired: 9 in]
                }
                frame 77 {
                  n155 = call <vilib>:"sit CONVERT DBL.vi"("Last Row"=w481, "Raw Data"=w482) -> ("Output"=→"Starboard VSP Direction":dbl)  [unwired: 9 in]
                }
              }
            }
          }
        }
        n156 = call <vilib>:"sit Check to Stop Client.vi"("error in (no error)"=w200) -> ("error out"=w201:errorcluster, "Stop?"=w199:bool)  [unwired: 2 in, 7 out]
        n157 = Wait (ms)(milliseconds to wait=u32 50) -> ()  [unwired: 1 out]
      }
      n158 = local write "SIT_Meta_Info"(w106) -> ()
      n159 = call <vilib>:"sit Merge SIT Client Errors.vi"("Bottom Loop Error"=w102, "Top Loop Error"=w100) -> ("Resulting Error"=w101:errorcluster)  [unwired: 9 out]
    }
    frame Error {
      # "User canceled target selection (or an error occurred on Init)...don't run the client"
      n160 = local write "SIT_Meta_Info"(w483) -> ()
    }
  }
  n161 = Current VI's Path() -> (path=w65:path)
  n162 = Current VI's Path() -> (path=w38:path)
  n163 = Current VI's Path() -> (path=w19:path)
  n164 = Current VI's Path() -> (path=w43:path)
  n165 = Strip Path(path=w65) -> (stripped path=w64:path)  [unwired: 1 out]
  n166 = Strip Path(path=w38) -> (stripped path=w37:path)  [unwired: 1 out]
  n167 = Strip Path(path=w19) -> (stripped path=w18:path)  [unwired: 1 out]
  n168 = Strip Path(path=w43) -> (stripped path=w42:path)  [unwired: 1 out]
  n169 = Build Path(base path=w64, name or relative path="model\\3D\\3dsboat55.wrl" ("Name")) -> (appended path=w61:path)
  n170 = call <vilib>:"Create Box.vi"("Color"=T12 {"Red"=0.0, "Green"=0.0, "Blue"=1.0, "Alpha"=1.0}, "Length Z"=sgl 6.5 ("Red"), "Length Y"=sgl 0.001 ("Red"), "Length X"=sgl 20.0 ("Red")) -> ("New Box Refnum"=w68:refnum<vi>)  [unwired: 6 in, 1 out]
  n171 = call <vilib>:"Create Object.vi"("Name"="Sea") -> ("Scene:New Object"=w69:refnum<vi>)  [unwired: 9 in, 1 out]
  n172 = Build Path(base path=w37, name or relative path="model\\3D\\3dsboatv2_yellow.wrl" ("Name")) -> (appended path=w34:path)
  n173 = Build Path(base path=w18, name or relative path="model\\3D\\target2.wrl" ("Name")) -> (appended path=w16:path)
  n174 = Build Path(base path=w42, name or relative path="model\\3D\\target2.wrl" ("Name")) -> (appended path=w40:path)
  n175 = call <vilib>:"Load VRML File.vi"("Path"=w61) -> ("Scene:Read Scene File"=w60:refnum<vi>)  [unwired: 9 in, 1 out]
  n176 = call <vilib>:"Create Object.vi"("Name"="Ship") -> ("Scene:New Object"=w62:refnum<vi>)  [unwired: 9 in, 1 out]
  n177 = call <vilib>:"Load VRML File.vi"("Path"=w34) -> ("Scene:Read Scene File"=w33:refnum<vi>)  [unwired: 9 in, 1 out]
  n178 = call <vilib>:"Create Object.vi"("Name"="Iceberg") -> ("Scene:New Object"=w35:refnum<vi>)  [unwired: 9 in, 1 out]
  n179 = call <vilib>:"Load VRML File.vi"("Path"=w16) -> ("Scene:Read Scene File"=w13:refnum<vi>)  [unwired: 9 in, 1 out]
  n180 = call <vilib>:"Load VRML File.vi"("Path"=w40) -> ("Scene:Read Scene File"=w39:refnum<vi>)  [unwired: 9 in, 1 out]
  n181 = invoke on="Invoke Node" class="SceneObject" method="Set Drawable"(reference=w69, "Drawable"=w68) -> (reference out=w57:refnum<vi>)  [unwired: 2 in, 3 out]
  n182 = while "Input Signal handeling from PS3 device" {
    tunnel: w77 -> [w544]
    tunnel: w76 -> [w543]
    tunnel: [w508] -> w72
    tunnel: [w509] -> w71
    stop <- w504 stop-if-true
    w510 = 0.1  # Step length
    w522 = 0.1  # Step length
    # "PS3 Signal updates every\n100 millisecond (10 Hz)\nmodify by editing number in\nblue box"
    # "Threshold preventing chattering"
    n183 = call-poly <vilib>:"Acquire Input Data.vi"("device ID"=w544, "error in (no error)"=w543) -> ("device ID"=w508:refnum<k1>, "axis info"=w540:T18, "button info"=w542:T19, "direction info"=w541:T20, "error out"=w509:errorcluster)  [unwired: 13 in]
    n184 = Unbundle By Name "Button info"(w542) -> ("button 1"=→"Square Button":bool, "button 2"=→"X Button":bool, "button 3"=→"Circle Button":bool, "button 4"=→"Triangle Button":bool, "button 7"=w502:bool, "button 8"=w503:bool, "button 9"=w526:bool, "button 10"=w514:bool, "button 11"=w525:bool, "button 12"=w513:bool)  [unwired: 2 out]
    "R2 Button" <- w502
    "L2 Button" <- w503
    "Direction Left" <- w526
    "Direction Down" <- w514
    "Direction Right" <- w525
    "Direction Up" <- w513
    n185 = Unbundle By Name "Direction info"(w541) -> ()  [unwired: 4 out]
    n186 = Unbundle By Name "Axis info"(w540) -> ("X axis"=w490:i32, "Y axis"=w539:i32, "Z axis"=w488:i32, "U axis"=w538:i32)  [unwired: 4 out]
    n187 = Negate(x=w538) -> (-x=w487:i32)
    n188 = Negate(x=w539) -> (-x=w489:i32)
    n189 = property on="Left Stick X" class="Slide (strict)"("Val(Sgnl)"=w490) -> ()  [unwired: 2 in, 2 out]
    n190 = property on="Right Stick X" class="Slide (strict)"("Val(Sgnl)"=w488) -> ()  [unwired: 2 in, 2 out]
    n191 = property on="Right Stick Y" class="Slide (strict)"("Val(Sgnl)"=w487) -> ()  [unwired: 2 in, 2 out]
    n192 = property on="Left Stick Y" class="Slide (strict)"("Val(Sgnl)"=w489) -> ()  [unwired: 2 in, 2 out]
    n193 = Boolean To (0,1)(Boolean=w502) -> (0, 1=w501:i16)
    n194 = Boolean To (0,1)(Boolean=w503) -> (0, 1=w498:i16)
    n195 = Negate(x=w501) -> (-x=w497:i16)
    n196 = Square(x=w488) -> (x^2=w495:i32)
    n197 = Square(x=w487) -> (x^2=w496:i32)
    n198 = Square(x=w490) -> (x^2=w493:i32)
    n199 = Square(x=w489) -> (x^2=w494:i32)
    n200 = property on="R2" class="DigNum (strict)"("Val(Sgnl)"=w497) -> ()  [unwired: 2 in, 2 out]
    n201 = property on="L2" class="DigNum (strict)"("Val(Sgnl)"=w498) -> ()  [unwired: 2 in, 2 out]
    n202 = feedback #1() -> (w531:bool)  [unwired: 1 in]
    n203 = feedback-in #1(w526) -> ()
    n204 = feedback #2() -> (w533:bool)  [unwired: 1 in]
    n205 = feedback-in #2(w525) -> ()
    n206 = feedback #3() -> (w519:bool)  [unwired: 1 in]
    n207 = feedback-in #3(w514) -> ()
    n208 = feedback #4() -> (w521:bool)  [unwired: 1 in]
    n209 = feedback-in #4(w513) -> ()
    n210 = Add(x=w493, y=w494) -> (x+y=w491:i32)
    n211 = Add(x=w495, y=w496) -> (x+y=w492:i32)
    n212 = Greater?(x=w526, y=w531) -> (0:w530:bool)
    n213 = Greater?(x=w525, y=w533) -> (0:w532:bool)
    n214 = Greater?(x=w514, y=w519) -> (0:w518:bool)
    n215 = Greater?(x=w513, y=w521) -> (0:w520:bool)
    n216 = Square Root(x=w491) -> (sqrt(x)=w486:dbl)
    n217 = Square Root(x=w492) -> (sqrt(x)=w485:dbl)
    n218 = call <vilib>:"Increment PtByPt.vi"("activate"=w530) -> ("counter"=w529:u32)  [unwired: 1 in, 1 out]
    n219 = call <vilib>:"Increment PtByPt.vi"("activate"=w532) -> ("counter"=w524:u32)  [unwired: 1 in, 1 out]
    n220 = call <vilib>:"Increment PtByPt.vi"("activate"=w518) -> ("counter"=w517:u32)  [unwired: 1 in, 1 out]
    n221 = call <vilib>:"Increment PtByPt.vi"("activate"=w520) -> ("counter"=w511:u32)  [unwired: 1 in, 1 out]
    n222 = To Double Precision Float(number=w529) -> (double precision float=w528:dbl)
    n223 = To Double Precision Float(number=w517) -> (double precision float=w516:dbl)
    n224 = call "Out of Range"("Operand 1"=w486) -> ("Result"=→"Left Joystick":dynamicdata)  [unwired: 9 in, 1 out]
    n225 = call "Out of Range"("Operand 1"=w485) -> ("Result"=→"Right Joystick":dynamicdata)  [unwired: 9 in, 1 out]
    n226 = Negate(x=w528) -> (-x=w527:dbl)
    n227 = Negate(x=w516) -> (-x=w512:dbl)
    n228 = Add(x=w527, y=w524) -> (x+y=w523:dbl)
    n229 = Add(x=w512, y=w511) -> (x+y=w515:dbl)
    n230 = Multiply(x=w523, y=w522) -> (x*y=w500:dbl)
    n231 = Multiply(x=w515, y=w510) -> (x*y=w499:dbl)
    n232 = property on="BT Slide Power Limiter" class="Slide (strict)"("Val(Sgnl)"=w500) -> ()  [unwired: 2 in, 2 out]
    n233 = property on="VSP Slide Speed" class="Slide (strict)"("Val(Sgnl)"=w499) -> ()  [unwired: 2 in, 2 out]
    n234 = property on="SIT_stopVI" class="Bool (strict)"() -> ("Value"=w504:bool)  [unwired: 2 in, 2 out]
    n235 = Wait (ms)(milliseconds to wait=u32 100) -> ()  [unwired: 1 out]
  }
  n236 = invoke on="Invoke Node" class="SceneObject" method="Object.Add Object"(reference=w62, "Child"=w60) -> (reference out=w56:refnum<vi>, "Child"=w55:refnum<vi>)  [unwired: 2 in, 2 out]
  n237 = invoke on="Invoke Node" class="SceneObject" method="Object.Add Object"(reference=w35, "Child"=w33) -> (reference out=w28:refnum<vi>, "Child"=w31:refnum<vi>)  [unwired: 2 in, 2 out]
  n238 = call <vilib>:"Create Object.vi"("Name"="DP waypoint") -> ("Scene:New Object"=w54:refnum<vi>)  [unwired: 9 in, 1 out]
  n239 = call <vilib>:"Create Object.vi"("Name"="Path marker") -> ("Scene:New Object"=w15:refnum<vi>)  [unwired: 9 in, 1 out]
  n240 = invoke on="3D Picture" class="SceneGraphDisp (strict)" method="Setup Camera"("Camera Position"=cluster{"X":sgl, "Y":sgl, "Z":sgl} {"X"=-15.0, "Y"=11.0, "Z"=0.0}, "Target"=cluster{"X":sgl, "Y":sgl, "Z":sgl} {"X"=0.0, "Y"=0.0, "Z"=0.0} ("Camera Position"), "Up Direction"=cluster{"X":sgl, "Y":sgl, "Z":sgl} {"X"=1.0, "Y"=0.0, "Z"=0.0} ("Camera Position")) -> ()  [unwired: 3 in, 6 out]
  n241 = call <vilib>:"Set Scale.vi"("Scale"=cluster{"X":sgl, "Y":sgl, "Z":sgl} {"X"=0.001, "Y"=0.001, "Z"=0.001} ("Initial Position"), "Scene Object"=w55) -> ("Scaled Object"=w27:refnum<vi>)  [unwired: 8 in, 1 out]
  n242 = call <vilib>:"Set Scale.vi"("Scale"=cluster{"X":sgl, "Y":sgl, "Z":sgl} {"X"=0.001, "Y"=0.001, "Z"=0.001} ("Initial Position"), "Scene Object"=w31) -> ("Scaled Object"=w25:refnum<vi>)  [unwired: 8 in, 1 out]
  n243 = invoke on="Invoke Node" class="SceneObject" method="Object.Add Object"(reference=w54, "Child"=w39) -> (reference out=w49:refnum<vi>, "Child"=w26:refnum<vi>)  [unwired: 2 in, 2 out]
  n244 = invoke on="Invoke Node" class="SceneObject" method="Object.Add Object"(reference=w15, "Child"=w13) -> (reference out=w10:refnum<vi>, "Child"=w9:refnum<vi>)  [unwired: 2 in, 2 out]
  n245 = invoke on="Invoke Node" class="SceneObject" method="Object.Add Object"(reference=w57, "Child"=w56) -> (reference out=w52:refnum<vi>)  [unwired: 2 in, 3 out]
  n246 = local write "SIT_stopVI"(w84) -> ()
  n247 = call <vilib>:"sit Clear Client.vi"("error in (no error)"=w90, "SIT Client Op Refs"=w86) -> ("error out"=w87:errorcluster)  [unwired: 9 out]
  n248 = call <vilib>:"sit Check to Stop Client.vi"("Reset Stop?"=TRUE ("Clear Item?"), "error in (no error)"=w87) -> ("error out"=w79:errorcluster)  [unwired: 1 in, 8 out]
  n249 = property on="3D Picture" class="SceneGraphDisp (strict)"("Background Color"=cluster{"X":sgl, "Y":sgl, "Z":sgl, "Z 2":sgl} {"X"=1.0, "Y"=1.0, "Z"=1.0, "Z 2"=1.0} ("Camera Position")) -> ()  [unwired: 2 in, 2 out]
  n250 = call <vilib>:"sit Check Run-Time System.vi"("error in"=w79) -> ("Run Time System?"=w78:bool)  [unwired: 10 out]
  n251 = Quit LabVIEW(quit? (T)=w78) -> ()
  n252 = invoke on="Invoke Node" class="SceneObject" method="Object.Add Object"(reference=w52, "Child"=w49) -> (reference out=w29:refnum<vi>)  [unwired: 2 in, 3 out]
  n253 = invoke on="Invoke Node" class="SceneObject" method="Object.Add Object"(reference=w29, "Child"=w28) -> (reference out=w12:refnum<vi>)  [unwired: 2 in, 3 out]
  n254 = call-poly <vilib>:"Close Input Device.vi"("error in (no error)"=w71, "device ID"=w72) -> ("error out"=w70:errorcluster)  [unwired: 8 in]
  n255 = property on="SIT_Run" class="Bool (strict)"() -> ("Value"=w20:bool)  [unwired: 2 in, 2 out]
  n256 = invoke on="Invoke Node" class="SceneObject" method="Object.Add Object"(reference=w12, "Child"=w10) -> (reference out=w11:refnum<vi>)  [unwired: 2 in, 3 out]
  n257 = call <vilib>:"General Error Handler.vi"("error in (no error)"=w70) -> ()  [unwired: 10 in, 5 out]
  n258 = case shown="True" w20 {
    frame False {
    }
    frame True {
      n259 = while {
        stop <- w546 stop-if-true
        # "Response charts DP"
        # "Response chart adds new point every\n100 milliseconds (10 Hz)\nmodify by editing blue box number"
        n260 = local read "DP eta_d N"() -> (w554:dbl)
        n261 = local read "DP eta N"() -> (w555:dbl)
        n262 = property on="DP eta Psi deg" class="DigNum (strict)"() -> ("Value"=w551:dbl)  [unwired: 2 in, 2 out]
        n263 = property on="DP eta_d Psi deg" class="DigNum (strict)"() -> ("Value"=w548:dbl)  [unwired: 2 in, 2 out]
        n264 = property on="DP eta E" class="DigNum (strict)"() -> ("Value"=w549:dbl)  [unwired: 2 in, 2 out]
        n265 = property on="DP eta_d E" class="DigNum (strict)"() -> ("Value"=w547:dbl)  [unwired: 2 in, 2 out]
        n266 = Bundle("Value"=w547, "Value"=w549) -> (→"DP Response E":cluster{"Value":dbl, "Value":dbl})  [unwired: 1 in]
        n267 = Bundle("Value"=w548, "Value"=w551) -> (→"DP Reponse Psi":cluster{"Value":dbl, "Value":dbl})  [unwired: 1 in]
        n268 = Bundle("DP eta_d N"=w554, "DP eta N"=w555) -> (→"DP Reponse N":cluster{"DP eta_d N":dbl, "DP eta N":dbl})  [unwired: 1 in]
        n269 = property on="SIT_Stop" class="Bool (strict)"() -> ("Value"=w546:bool)  [unwired: 2 in, 2 out]
        n270 = Wait (ms)(milliseconds to wait=u32 100) -> ()  [unwired: 1 out]
      }
    }
  }
  n271 = while {
    tunnel: w11 -> [w615]
    tunnel: w27 -> [w621]
    tunnel: w26 -> [w619]
    tunnel: w25 -> [w587]
    tunnel: w9 -> [w557]
    stop <- w614 stop-if-true
    # "yaw -> rotate around \ny-axis of boat model"
    # "3D display updates every\n100 miliseconds (10 Hz)\nmodify by editing the\nblue box number"
    # "yaw -> rotate around \ny-axis of  model"
    # "xzy due to boat bottom to top direction is along y-axis"
    # "yaw -> rotate around \ny-axis of boat model"
    # "yaw -> rotate around \ny-axis of model"
    # "xzy due to boat bottom to top direction is along y-axis"
    n272 = Not(x="Show DP Marker") -> (.not. x?=w578:bool)
    n273 = property on="CSE1 x-position [m]" class="DigNum (strict)"() -> ("Value"=w611:dbl)  [unwired: 2 in, 2 out]
    n274 = property on="CSE1 z-position [m]" class="DigNum (strict)" props=["Value"]() -> ()  [unwired: 2 in, 3 out]
    n275 = property on="CSE1 y-position [m]" class="DigNum (strict)"() -> ("Value"=w608:dbl)  [unwired: 2 in, 2 out]
    n276 = property on="Path x_d" class="DigNum (strict)"() -> ("Value"=w565:dbl)  [unwired: 2 in, 2 out]
    n277 = property on="Path y_d" class="DigNum (strict)"() -> ("Value"=w563:dbl)  [unwired: 2 in, 2 out]
    n278 = Boolean To (0,1)(Boolean=w578) -> (0, 1=w580:i16)
    n279 = Not(x="Show Path Marker") -> (.not. x?=w569:bool)
    n280 = Not(x="Show CSEI") -> (.not. x?=w604:bool)
    n281 = property on="Iceberg x-position" class="DigNum (strict)"() -> ("Value"=w595:dbl)  [unwired: 2 in, 2 out]
    n282 = property on="Iceberg z-position" class="DigNum (strict)" props=["Value"]() -> ()  [unwired: 2 in, 3 out]
    n283 = property on="Iceberg y-position" class="DigNum (strict)"() -> ("Value"=w592:dbl)  [unwired: 2 in, 2 out]
    n284 = Boolean To (0,1)(Boolean=w569) -> (0, 1=w571:i16)
    n285 = Boolean To (0,1)(Boolean=w604) -> (0, 1=w607:i16)
    n286 = Multiply(x=w608, y=1) -> (x*y=w609:dbl)
    n287 = Multiply(x=w563, y=1) -> (x*y=w560:dbl)
    n288 = Multiply(x=w580, y=-1) -> (x*y=w575:i32)
    n289 = Not(x="Show Iceberg") -> (.not. x?=w589:bool)
    n290 = Multiply(x=w611, y=1) -> (x*y=w612:dbl)
    n291 = Multiply(x=w565, y=1) -> (x*y=w561:dbl)
    n292 = Multiply(x="DP eta_d_Psi [deg]", y=3.141592653589793) -> (x*y=w583:dbl)
    n293 = Boolean To (0,1)(Boolean=w589) -> (0, 1=w591:i16)
    n294 = Multiply(x=w571, y=-1) -> (x*y=w562:i32)
    n295 = Multiply(x=w592, y=1) -> (x*y=w593:dbl)
    n296 = Bundle("DP eta_d_N [m]"="DP eta_d_N [m]", w575, "DP eta_d_E [m]"="DP eta_d_E [m]") -> (w574:T21)  [unwired: 1 in]
    n297 = Multiply(x=w595, y=1) -> (x*y=w596:dbl)
    n298 = Multiply(x=w607, y=-1) -> (x*y=w603:i32)
    n299 = Bundle(w561, w562, w560) -> (w568:cluster{dbl, i32, dbl})  [unwired: 1 in]
    n300 = Divide(x=w583, y=180) -> (x/y=w581:dbl)
    "Ind eta_d_Psi [rad]" <- w581
    n301 = Bundle(w612, w603, w609) -> (w620:cluster{dbl, i32, dbl})  [unwired: 1 in]
    n302 = call <vilib>:"Set Translation.vi"("Translation"=w574, "Scene Object"=w619) -> ("Translated Object"=w618:refnum<vi>)  [unwired: 8 in, 1 out]
    n303 = Multiply(x=w591, y=-1) -> (x*y=w588:i32)
    n304 = call <vilib>:"Set Translation.vi"("Translation"=w568, "Scene Object"=w557) -> ("Translated Object"=w556:refnum<vi>)  [unwired: 8 in, 1 out]
    n305 = Bundle(w596, w588, w593) -> (w598:cluster{dbl, i32, dbl})  [unwired: 1 in]
    n306 = property on="Path psi_d" class="DigNum (strict)"() -> ("Value"=w559:dbl)  [unwired: 2 in, 2 out]
    n307 = Negate(x=w581) -> (-x=w616:dbl)
    n308 = property on="CSE1 pitch [rad]" class="DigNum (strict)" props=["Value"]() -> ()  [unwired: 2 in, 3 out]
    n309 = property on="CSE1 yaw [rad]" class="DigNum (strict)"() -> ("Value"=w623:dbl)  [unwired: 2 in, 2 out]
    n310 = property on="CSE1 roll [rad]" class="DigNum (strict)" props=["Value"]() -> ()  [unwired: 2 in, 3 out]
    n311 = call <vilib>:"Set Translation.vi"("Translation"=w620, "Scene Object"=w621) -> ("Translated Object"=w625:refnum<vi>)  [unwired: 8 in, 1 out]
    n312 = Negate(x=w559) -> (-x=w558:dbl)
    n313 = call <vilib>:"Set Rotation.vi"("Angle"=w616, "Axis"=cluster{"X":sgl, "Y":sgl, "Z":sgl} {"X"=0.0, "Y"=1.0, "Z"=0.0} ("Camera Position"), "Scene Object"=w618) -> ()  [unwired: 7 in, 2 out]
    n314 = property on="Iceberg pitch" class="DigNum (strict)" props=["Value"]() -> ()  [unwired: 2 in, 3 out]
    n315 = property on="Iceberg yaw" class="DigNum (strict)"() -> ("Value"=w600:dbl)  [unwired: 2 in, 2 out]
    n316 = property on="Iceberg roll" class="DigNum (strict)" props=["Value"]() -> ()  [unwired: 2 in, 3 out]
    n317 = Negate(x=w623) -> (-x=w622:dbl)
    n318 = call <vilib>:"Set Translation.vi"("Translation"=w598, "Scene Object"=w587) -> ("Translated Object"=w602:refnum<vi>)  [unwired: 8 in, 1 out]
    n319 = call <vilib>:"Set Rotation.vi"("Angle"=w558, "Axis"=cluster{"X":sgl, "Y":sgl, "Z":sgl} {"X"=0.0, "Y"=1.0, "Z"=0.0} ("Camera Position"), "Scene Object"=w556) -> ()  [unwired: 7 in, 2 out]
    n320 = property on="SIT_stopVI" class="Bool (strict)"() -> ("Value"=w614:bool)  [unwired: 2 in, 2 out]
    n321 = Negate(x=w600) -> (-x=w599:dbl)
    n322 = Wait (ms)(milliseconds to wait=u32 100) -> ()  [unwired: 1 out]
    n323 = call <vilib>:"Set Rotation.vi"("Angle"=w622, "Axis"=cluster{"X":sgl, "Y":sgl, "Z":sgl} {"X"=0.0, "Y"=1.0, "Z"=0.0} ("Camera Position"), "Scene Object"=w625) -> ()  [unwired: 7 in, 2 out]
    n324 = call <vilib>:"Set Rotation.vi"("Angle"=w599, "Axis"=cluster{"X":sgl, "Y":sgl, "Z":sgl} {"X"=0.0, "Y"=1.0, "Z"=0.0} ("Camera Position"), "Scene Object"=w602) -> ()  [unwired: 7 in, 2 out]
    "3D Picture" <- w615
  }
